vi "RT Main.vi"() -> ()   [LabVIEW 2013]
uses:
  SubVIs/growbed_states.ctl
  SubVIs/fishtank_level_states.ctl
  SubVIs/fishtank_states.ctl
  <vilib>/Platform/TimedLoop/XDataNode/timing_clust.ctl
  <vilib>/Platform/TimedLoop/XDataNode/nitl_modes.ctl
  <vilib>/Platform/TimedLoop/XDataNode/wakeup.ctl
  SubVIs/FGV_enum.ctl
  <vilib>/rvi/interface/common/niFpgaWaitOnOcc.vi
  <vilib>/FPGAPlugInAG/myRIO-1900/niLvFpga_Open_myRIO-1900.vi
  <vilib>/rvi/interface/common/dynamic/niFpgaDynamicAddResources.vi
  <vilib>/Utility/error.llb/Error Cluster From Error Code.vi
  <vilib>/rvi/errors/niLvFpgaAdjustHostInterfaceError.vi
  <vilib>/FPGAPlugInAG/Dynamic/niLvFpga_Run_Dynamic.vi
  <vilib>/FPGAPlugInAG/Dynamic/niLvFpga_Close_Dynamic.vi
  <vilib>/rvi/interface/nirviOpenFPGA/nirviOpenFPGA.xnode
  FPGA Bitfiles/myRIOAquaponics_FPGATarget_Main(FPGA)_Pb0EBwUZ3xI.lvbitx
  <vilib>/rvi/interface/nirviReadWriteControl/nirviReadWriteControl.xnode
  <vilib>/Platform/TimedLoop/XDataNode/XDataNode.xnode
  <vilib>/rvi/interface/nirviMethod/nirviMethod.xnode
  <vilib>/rvi/interface/nirviCloseFPGA/nirviCloseFPGA.xnode
  <vilib>/Platform/TimedLoop/XDataNode/XDNodeRunTimeDep.lvlib
  NiFpgaLv.dll
  <vilib>/rvi/interface/Simulation/niFpgaSimulationCallBeginRW.vi
  <vilib>/rvi/errors/niLvFpgaMergeErrorWithErrorCode.vi
  <vilib>/FPGAPlugInAG/Dynamic/niLvFpga_ConfigureFifo_Dynamic.vi
  <vilib>/FPGAPlugInAG/Dynamic/niLvFpga_StartFifo_Dynamic.vi
  <vilib>/FPGAPlugInAG/Dynamic/niLvFpga_ReadFifo_Dynamic.vi
  <vilib>/FPGAPlugInAG/Dynamic/niLvFpga_StopFifo_Dynamic.vi
panel:
  out "Fishtank States - Temperature":T1=enum."Low Temperature (Heater ON)"
  out "pH Signal":dbl[](graph)=[0.029296875, 0.0244140625, 0.0244140625, 0.0244140625, 0.01953125, 0.029296875, 0.0244140625, 0.0244140625, 0.0244140625, 0.0244140625, 0.029296875, 0.0244140625, 0.0244140625, 0.029296875, 0.0244140625, 0.029296875, 0.0244140625, 0.0244140625, 0.0244140625, 0.029296875, 0.029296875, 0.0244140625, 0.0244140625, 0.0244140625, 0.029296875, 0.0244140625, 0.0244140625, 0.029296875, 0.0244140625, 0.029296875, 0.029296875, 0.0244140625, 0.029296875, 0.029296875, 0.0244140625, 0.0244140625, 0.0244140625, 0.029296875, 0.029296875, 0.0244140625, 0.029296875, 0.0244140625, 0.029296875, 0.0244140625, 0.029296875, 0.029296875, 0.029296875, 0.0244140625, 0.0244140625, 0.0244140625, 0.0341796875, 0.0244140625, 0.029296875, 0.0244140625, 0.0244140625, 0.029296875, 0.029296875, 0.0341796875, 0.0341796875, 0.0390625, 0.0439453125, 0.0390625, 0.0341796875, 0.0439453125, 0.0439453125, 0.0390625, 0.0439453125, 0.0390625, 0.048828125, 0.0439453125, 0.0390625, 0.0390625, 0.0390625, 0.0439453125, 0.0439453125, 0.0341796875, 0.0439453125, 0.048828125, 0.0390625, 0.048828125, 0.0439453125, 0.048828125, 0.0439453125, 0.0390625, 0.0439453125, 0.0439453125, 0.0439453125, 0.0439453125, 0.0390625, 0.0439453125, 0.0439453125, 0.0439453125, 0.0439453125, 0.0439453125, 0.048828125, 0.048828125, 0.0390625, 0.0439453125, 0.0439453125, 0.0439453125, 0.048828125, 0.0439453125, 0.048828125, 0.048828125, 0.0439453125, 0.048828125, 0.048828125, 0.048828125, 0.048828125, 0.0439453125, 0.048828125, 0.048828125, 0.0390625, 0.048828125, 0.048828125, 0.048828125, 0.048828125, 0.0439453125, 0.048828125, 0.048828125, 0.0439453125, 0.0537109375, 0.048828125, 0.0439453125, 0.048828125, 0.048828125, 0.048828125, 0.0537109375, 0.0439453125, 0.0537109375, 0.048828125, 0.0439453125, 0.048828125, 0.048828125, 0.0439453125, 0.048828125, 0.0439453125, 0.048828125, 0.048828125, 0.048828125, 0.0537109375, 0.048828125, 0.0439453125, 0.0537109375, 0.048828125, 0.0439453125, 0.048828125, 0.0537109375, 0.048828125, 0.0537109375, 0.0439453125, 0.0537109375, 0.048828125, 0.0439453125, 0.05859375, 0.048828125, 0.0439453125, 0.048828125, 0.048828125, 0.048828125, 0.048828125, 0.048828125, 0.048828125, 0.048828125, 0.0439453125, 0.048828125, 0.048828125, 0.048828125, 0.0537109375, 0.048828125, 0.048828125, 0.05859375, 0.048828125, 0.0390625, 0.0537109375, 0.048828125, 0.0439453125, 0.048828125, 0.048828125, 0.048828125, 0.0439453125, 0.048828125, 0.048828125, 0.048828125, 0.0439453125, 0.048828125, 0.048828125, 0.048828125, 0.0537109375, 0.048828125, 0.0439453125, 0.048828125, 0.048828125, 0.048828125, 0.0439453125, 0.048828125, 0.048828125, 0.0439453125, 0.048828125, 0.0537109375, 0.048828125, 0.048828125, 0.048828125, 0.048828125, 0.048828125, 0.0439453125, 0.0537109375, 0.048828125, 0.048828125, 0.0439453125, 0.048828125, 0.048828125, 0.048828125, 0.0537109375, 0.048828125, 0.048828125, 0.0439453125, 0.048828125, 0.048828125, 0.048828125, 0.048828125, 0.0537109375, 0.048828125, 0.0439453125, 0.048828125, 0.048828125, 0.048828125, 0.048828125, 0.048828125, 0.0537109375, 0.048828125, 0.048828125, 0.0390625, 0.048828125, 0.048828125, 0.048828125, 0.048828125, 0.048828125, 0.048828125, 0.0439453125, 0.048828125, 0.048828125, 0.048828125, 0.048828125, 0.0439453125, 0.048828125, 0.0537109375, 0.0439453125, 0.0537109375, 0.048828125, 0.048828125, 0.048828125, 0.0439453125, 0.0537109375, 0.0537109375, 0.0439453125, 0.048828125, 0.048828125, 0.048828125, 0.048828125, 0.048828125, 0.0537109375, 0.048828125, 0.0439453125, 0.0439453125, 0.048828125, 0.0537109375, 0.048828125, 0.0439453125, 0.0439453125, 0.048828125, 0.048828125, 0.048828125, 0.048828125, 0.0537109375, 0.048828125, 0.048828125, 0.0439453125, 0.048828125, 0.0537109375, 0.048828125, 0.0439453125, 0.048828125, 0.048828125, 0.048828125, 0.048828125, 0.0439453125, 0.048828125, 0.048828125, 0.0390625, 0.048828125, 0.0439453125, 0.0439453125, 0.048828125, 0.0439453125, 0.048828125, 0.048828125, 0.0439453125, 0.048828125, 0.0439453125, 0.0439453125, 0.048828125, 0.048828125, 0.048828125, 0.0439453125, 0.048828125, 0.048828125, 0.048828125, 0.0537109375, 0.0439453125, 0.048828125, 0.0439453125, 0.048828125, 0.048828125, 0.0439453125, 0.048828125, 0.0439453125, 0.048828125, 0.048828125, 0.0390625, 0.048828125, 0.0439453125, 0.048828125, 0.048828125, 0.0390625, 0.048828125, 0.048828125, 0.0439453125, 0.0439453125, 0.0439453125, 0.048828125, 0.0439453125, 0.0439453125, 0.0439453125, 0.0390625, 0.048828125, 0.0439453125, 0.0439453125, 0.048828125, 0.0390625, 0.048828125, 0.0390625, 0.0439453125, 0.048828125, 0.0390625, 0.048828125, 0.0390625, 0.0390625, 0.0439453125, 0.0439453125, 0.048828125, 0.0390625, 0.0439453125, 0.0439453125, 0.0439453125, 0.0439453125, 0.0439453125, 0.048828125, 0.0390625, 0.0439453125, 0.0439453125, 0.0390625, 0.048828125, 0.0341796875, 0.0390625, 0.0439453125, 0.0439453125, 0.0439453125, 0.0390625, 0.048828125, 0.0439453125, 0.0390625, 0.0439453125, 0.0439453125, 0.0439453125, 0.0341796875, 0.0390625, 0.0439453125, 0.0439453125, 0.0439453125, 0.0390625, 0.048828125, 0.0439453125, 0.0390625, 0.048828125, 0.0390625, 0.0439453125, 0.0390625, 0.0439453125, 0.0439453125, 0.0390625, 0.0390625, 0.0390625, 0.0439453125, 0.0390625, 0.0439453125, 0.0439453125, 0.0439453125, 0.0439453125, 0.0390625, 0.0390625, 0.0439453125, 0.0439453125, 0.0439453125, 0.0390625, 0.0439453125, 0.0439453125, 0.0390625, 0.0439453125, 0.0390625, 0.0390625, 0.0341796875, 0.0439453125, 0.0439453125, 0.0390625, 0.0439453125, 0.0390625, 0.0439453125, 0.0390625, 0.0439453125, 0.0439453125, 0.0341796875, 0.0439453125, 0.0439453125, 0.0390625, 0.0439453125, 0.0390625, 0.0439453125, 0.0439453125, 0.0439453125, 0.0439453125, 0.0390625, 0.0390625, 0.0341796875, 0.0390625, 0.0439453125, 0.0390625, 0.0439453125, 0.0341796875, 0.0439453125, 0.048828125, 0.0390625, 0.0390625, 0.0341796875, 0.0390625, 0.0439453125, 0.0390625, 0.0390625, 0.0390625, 0.0390625, 0.0390625, 0.0439453125, 0.0439453125, 0.0390625, 0.0390625, 0.0390625, 0.0439453125, 0.0390625, 0.0341796875, 0.0439453125, 0.0439453125, 0.0439453125, 0.0390625, 0.0390625, 0.0390625, 0.0439453125, 0.0439453125, 0.0439453125, 0.0390625, 0.0390625, 0.0439453125, 0.0390625, 0.0439453125, 0.0439453125, 0.0439453125, 0.0390625, 0.0439453125, 0.0390625, 0.0390625, 0.0439453125, 0.0439453125, 0.0439453125, 0.0390625, 0.0439453125, 0.048828125, 0.0390625, 0.0390625, 0.0390625, 0.0390625, 0.0439453125, 0.0439453125, 0.0439453125, 0.048828125, 0.0390625, 0.0390625, 0.0390625, 0.0439453125, 0.0439453125, 0.0439453125, 0.0390625, 0.0390625, 0.0439453125, 0.0439453125, 0.0439453125, 0.0439453125, 0.0439453125, 0.0439453125, 0.0390625, 0.0390625, 0.0439453125, 0.0439453125, 0.0439453125, 0.0439453125, 0.0439453125, 0.0439453125, 0.0390625, 0.0390625, 0.0439453125, 0.0439453125, 0.0390625, 0.0439453125, 0.0439453125, 0.0390625, 0.0439453125, 0.0390625, 0.0439453125, 0.0439453125, 0.0390625, 0.0439453125, 0.0439453125, 0.0439453125, 0.0439453125, 0.0390625, 0.0439453125, 0.0439453125, 0.0439453125, 0.0439453125, 0.0439453125, 0.0439453125, 0.0439453125, 0.0390625, 0.0439453125, 0.0439453125, 0.0390625, 0.0439453125, 0.048828125, 0.0390625, 0.0439453125, 0.0439453125, 0.0390625, 0.0439453125, 0.0390625, 0.0439453125, 0.048828125, 0.0390625, 0.0390625, 0.048828125, 0.0390625, 0.0439453125, 0.048828125, 0.0390625, 0.0390625, 0.0390625, 0.0439453125, 0.0439453125, 0.0390625, 0.0390625, 0.0439453125, 0.0390625, 0.0390625, 0.048828125, 0.0439453125, 0.0390625, 0.0439453125, 0.0390625, 0.0390625, 0.0390625, 0.0390625, 0.048828125, 0.0390625, 0.0390625, 0.0439453125, 0.0390625, 0.0390625, 0.0439453125, 0.0390625, 0.048828125, 0.0439453125, 0.0439453125, 0.0390625, 0.0439453125, 0.0390625, 0.0390625, 0.0439453125, 0.0390625, 0.0439453125, 0.0390625, 0.0439453125, 0.0439453125, 0.0341796875, 0.0439453125, 0.0439453125, 0.0439453125, 0.0390625, 0.0439453125, 0.0390625, 0.0439453125, 0.0439453125, 0.0439453125, 0.0390625, 0.0390625, 0.0439453125, 0.0390625, 0.0390625, 0.0439453125, 0.0439453125, 0.0390625, 0.0439453125, 0.0439453125, 0.0439453125, 0.0390625, 0.0390625, 0.0439453125, 0.0390625, 0.0390625, 0.0439453125, 0.0439453125, 0.0439453125, 0.0439453125, 0.0439453125, 0.0439453125, 0.0390625, 0.0390625, 0.0439453125, 0.0439453125, 0.0390625, 0.0439453125, 0.0439453125, 0.0390625, 0.0439453125, 0.048828125, 0.0390625, 0.0439453125, 0.0390625, 0.0439453125, 0.0439453125, 0.0439453125, 0.0439453125, 0.0439453125, 0.0439453125, 0.0439453125, 0.0390625, 0.0439453125, 0.0439453125, 0.0390625, 0.0390625, 0.0439453125, 0.0439453125, 0.0390625, 0.0390625, 0.0390625, 0.0439453125, 0.0439453125, 0.0390625, 0.048828125, 0.0390625, 0.0390625, 0.0390625, 0.0439453125, 0.0439453125, 0.0439453125, 0.0439453125, 0.048828125, 0.0439453125, 0.0439453125, 0.0390625, 0.0390625, 0.0439453125, 0.0439453125, 0.0390625, 0.0439453125, 0.0390625, 0.0439453125, 0.0439453125, 0.0390625, 0.0439453125, 0.0439453125, 0.0390625, 0.0390625, 0.0439453125, 0.0439453125, 0.0390625, 0.0390625, 0.0390625, 0.0439453125, 0.0390625, 0.0390625, 0.0439453125, 0.0390625, 0.0390625, 0.0439453125, 0.0390625, 0.0390625, 0.048828125, 0.0439453125, 0.0439453125, 0.0390625, 0.0390625, 0.048828125, 0.0390625, 0.0390625, 0.0390625, 0.0439453125, 0.0439453125, 0.0439453125, 0.0341796875, 0.0390625, 0.0439453125, 0.0439453125, 0.0439453125, 0.0390625, 0.0390625, 0.0439453125, 0.0390625, 0.0439453125, 0.0390625, 0.0390625, 0.0390625, 0.0439453125, 0.0390625, 0.0439453125, 0.0390625, 0.0390625, 0.0439453125, 0.0439453125, 0.0390625, 0.0439453125, 0.0390625, 0.0390625, 0.0390625, 0.0390625, 0.0390625, 0.0439453125, 0.0390625, 0.0439453125, 0.0341796875, 0.0390625, 0.0439453125, 0.0390625, 0.0390625, 0.0390625, 0.0390625, 0.0390625, 0.0439453125, 0.0390625, 0.0439453125, 0.0390625, 0.0390625, 0.0439453125, 0.0390625, 0.0390625, 0.0390625, 0.0390625, 0.0390625, 0.0390625, 0.0390625, 0.0439453125, 0.0439453125, 0.0390625, 0.0439453125, 0.0390625, 0.0390625, 0.0390625, 0.0341796875, 0.0390625, 0.0439453125, 0.0390625, 0.0439453125, 0.0390625, 0.0439453125, 0.0439453125, 0.0390625, 0.0341796875, 0.0439453125, 0.0341796875, 0.0390625, 0.0439453125, 0.0439453125, 0.0390625, 0.0439453125, 0.0390625, 0.0390625, 0.0390625, 0.0390625, 0.0390625, 0.0390625, 0.0390625, 0.0390625, 0.0390625, 0.0439453125, 0.0390625, 0.0390625, 0.0439453125, 0.0390625, 0.0390625, 0.0390625, 0.0390625, 0.0341796875, 0.0390625, 0.0390625, 0.0390625, 0.0439453125, 0.0390625, 0.0390625, 0.0439453125, 0.0390625, 0.0390625, 0.0390625, 0.0390625, 0.0390625, 0.0341796875, 0.0341796875, 0.0390625, 0.0390625, 0.0390625, 0.0390625, 0.0341796875, 0.0390625, 0.0439453125, 0.0341796875, 0.0390625, 0.0390625, 0.0390625, 0.0390625, 0.0390625, 0.0390625, 0.0390625, 0.0341796875, 0.0390625, 0.0439453125, 0.0439453125, 0.0390625, 0.0390625, 0.0341796875, 0.0390625, 0.0390625, 0.0390625, 0.0390625, 0.0341796875, 0.0341796875, 0.0439453125, 0.0390625, 0.0390625, 0.0341796875, 0.0341796875, 0.0439453125, 0.0341796875, 0.0390625, 0.0390625, 0.0390625, 0.0390625, 0.0341796875, 0.0390625, 0.0439453125, 0.0390625, 0.0390625, 0.0390625, 0.0341796875, 0.0390625, 0.0390625, 0.0390625, 0.0341796875, 0.0390625, 0.0390625, 0.0390625, 0.0439453125, 0.0341796875, 0.0390625, 0.0341796875, 0.0341796875, 0.0390625, 0.029296875, 0.0244140625, 0.0244140625, 0.0244140625, 0.01953125, 0.029296875, 0.01953125, 0.01953125, 0.0244140625, 0.01953125, 0.029296875, 0.0146484375, 0.01953125, 0.029296875, 0.01953125, 0.0244140625, 0.01953125, 0.01953125, 0.0244140625, 0.01953125, 0.01953125, 0.0244140625, 0.01953125, 0.0244140625, 0.01953125, 0.0146484375, 0.0244140625, 0.01953125, 0.01953125, 0.01953125, 0.0146484375, 0.01953125, 0.0146484375, 0.01953125, 0.01953125, 0.01953125, 0.0244140625, 0.0146484375, 0.0146484375, 0.01953125, 0.0146484375, 0.01953125, 0.01953125, 0.0146484375, 0.01953125, 0.0146484375, 0.01953125, 0.0146484375, 0.0146484375, 0.0244140625, 0.0146484375, 0.009765625, 0.01953125, 0.0146484375, 0.01953125, 0.0146484375, 0.0146484375, 0.0244140625, 0.009765625, 0.009765625, 0.01953125, 0.0146484375, 0.0146484375, 0.0146484375, 0.0146484375, 0.01953125, 0.0146484375, 0.009765625, 0.01953125, 0.009765625, 0.009765625, 0.01953125, 0.009765625, 0.01953125, 0.01953125, 0.0146484375, 0.01953125, 0.009765625, 0.0146484375, 0.01953125, 0.009765625, 0.0146484375, 0.0146484375, 0.009765625, 0.01953125, 0.009765625, 0.009765625, 0.0146484375, 0.009765625, 0.0146484375, 0.01953125, 0.009765625, 0.0146484375, 0.0146484375, 0.009765625, 0.0146484375, 0.0146484375, 0.0146484375, 0.0146484375, 0.009765625, 0.009765625, 0.01953125, 0.009765625, 0.0146484375, 0.0146484375, 0.009765625, 0.0146484375, 0.0146484375, 0.0146484375, 0.01953125, 0.009765625, 0.0146484375, 0.0146484375, 0.009765625, 0.009765625, 0.01953125, 0.009765625, 0.009765625, 0.0146484375, 0.009765625, 0.0146484375, 0.01953125, 0.009765625, 0.0146484375, 0.0146484375, 0.0146484375, 0.01953125, 0.0146484375, 0.0146484375, 0.01953125, 0.0048828125, 0.0146484375, 0.01953125, 0.009765625, 0.009765625, 0.01953125, 0.009765625, 0.0146484375, 0.0146484375, 0.009765625, 0.0146484375, 0.0146484375, 0.009765625, 0.01953125, 0.009765625, 0.0146484375, 0.0146484375, 0.009765625, 0.0146484375, 0.01953125, 0.009765625, 0.0146484375, 0.0146484375, 0.009765625, 0.01953125, 0.0146484375, 0.0146484375, 0.01953125, 0.009765625, 0.009765625, 0.01953125, 0.009765625, 0.0146484375, 0.01953125, 0.009765625, 0.0146484375, 0.0146484375, 0.0146484375, 0.01953125, 0.0048828125, 0.009765625, 0.01953125, 0.009765625, 0.01953125, 0.0146484375, 0.0146484375, 0.01953125, 0.0048828125, 0.009765625, 0.0146484375, 0.009765625, 0.0146484375, 0.0146484375, 0.009765625, 0.0146484375, 0.0146484375, 0.0146484375, 0.01953125, 0.0146484375, 0.009765625, 0.01953125, 0.009765625, 0.0146484375, 0.0244140625, 0.0146484375, 0.0146484375, 0.0146484375, 0.0048828125, 0.01953125, 0.0146484375, 0.009765625, 0.009765625, 0.009765625, 0.0146484375, 0.009765625, 0.009765625, 0.0146484375, 0.0146484375, 0.0146484375, 0.009765625, 0.0146484375, 0.0146484375, 0.0146484375, 0.0146484375, 0.0146484375, 0.01953125, 0.01953125, 0.009765625, 0.0146484375, 0.01953125, 0.0146484375, 0.0146484375, 0.0146484375, 0.0146484375, 0.0146484375, 0.009765625, 0.01953125, 0.0146484375, 0.0146484375, 0.01953125, 0.009765625, 0.009765625, 0.0146484375, 0.009765625, 0.0146484375, 0.009765625, 0.009765625, 0.01953125, 0.009765625, 0.0146484375, 0.0146484375, 0.0146484375, 0.01953125, 0.0146484375, 0.01953125, 0.0244140625, 0.0244140625, 0.01953125, 0.01953125, 0.01953125, 0.01953125, 0.0244140625, 0.0244140625, 0.01953125, 0.01953125, 0.0244140625, 0.0244140625, 0.0244140625, 0.01953125, 0.01953125, 0.0244140625, 0.0244140625, 0.0244140625, 0.0146484375, 0.01953125, 0.0244140625, 0.01953125, 0.0244140625, 0.0146484375, 0.01953125, 0.0244140625, 0.0244140625, 0.0244140625, 0.01953125, 0.01953125, 0.01953125, 0.0244140625, 0.029296875, 0.01953125, 0.0244140625, 0.01953125, 0.0244140625, 0.029296875, 0.01953125, 0.0244140625, 0.01953125, 0.0244140625, 0.029296875, 0.01953125, 0.0244140625, 0.0244140625, 0.01953125, 0.01953125, 0.01953125, 0.0244140625, 0.0244140625, 0.01953125, 0.0244140625, 0.0244140625, 0.0244140625, 0.0146484375, 0.01953125, 0.0244140625, 0.0244140625, 0.0244140625, 0.01953125, 0.01953125, 0.0244140625, 0.01953125, 0.0244140625, 0.01953125, 0.0244140625, 0.0244140625, 0.01953125, 0.0244140625, 0.01953125, 0.01953125, 0.0146484375, 0.01953125, 0.0244140625, 0.0244140625, 0.0244140625, 0.01953125, 0.0244140625, 0.01953125, 0.0244140625, 0.0244140625, 0.01953125, 0.0244140625, 0.01953125, 0.01953125, 0.0244140625, 0.0244140625, 0.0244140625, 0.0244140625, 0.0244140625, 0.0244140625, 0.01953125, 0.0244140625, 0.01953125, 0.0244140625, 0.01953125, 0.01953125, 0.01953125, 0.0244140625, 0.029296875, 0.01953125, 0.0244140625, 0.01953125, 0.01953125, 0.0244140625, 0.0244140625, 0.0244140625, 0.0146484375, 0.01953125, 0.01953125, 0.029296875, 0.0244140625, 0.01953125, 0.0244140625, 0.0244140625, 0.0244140625, 0.0244140625, 0.01953125, 0.029296875, 0.01953125, 0.01953125, 0.0244140625, 0.0244140625, 0.0244140625, 0.01953125, 0.0146484375, 0.01953125, 0.0244140625, 0.029296875, 0.0146484375, 0.0244140625, 0.0244140625, 0.0244140625, 0.0244140625, 0.01953125, 0.029296875, 0.01953125, 0.01953125, 0.029296875, 0.01953125, 0.029296875, 0.01953125, 0.01953125, 0.0244140625, 0.01953125, 0.0244140625, 0.01953125, 0.01953125, 0.0244140625, 0.0244140625, 0.01953125, 0.01953125, 0.0244140625, 0.01953125, 0.0244140625, 0.0244140625, 0.01953125, 0.01953125, 0.0244140625, 0.0244140625, 0.0244140625, 0.01953125, 0.01953125, 0.0244140625, 0.0244140625, 0.0244140625, 0.0244140625, 0.01953125, 0.01953125, 0.0244140625, 0.0244140625, 0.0244140625, 0.01953125, 0.01953125, 0.0244140625, 0.0244140625, 0.0244140625, 0.0244140625, 0.01953125, 0.01953125, 0.01953125, 0.01953125, 0.029296875, 0.0244140625, 0.01953125, 0.0244140625, 0.01953125, 0.0244140625, 0.01953125, 0.0146484375, 0.01953125, 0.0244140625, 0.0244140625, 0.0244140625, 0.0244140625, 0.0244140625, 0.01953125, 0.0244140625, 0.01953125, 0.01953125, 0.0244140625, 0.01953125, 0.0244140625, 0.01953125, 0.0244140625, 0.0244140625, 0.01953125, 0.0244140625, 0.01953125, 0.01953125, 0.0244140625, 0.0146484375, 0.01953125, 0.0244140625, 0.0244140625, 0.01953125, 0.0244140625, 0.0244140625, 0.0244140625, 0.01953125, 0.0146484375, 0.0244140625, 0.0244140625, 0.01953125, 0.01953125, 0.01953125, 0.01953125, 0.0244140625, 0.0244140625, 0.0244140625, 0.0244140625, 0.01953125, 0.01953125, 0.01953125, 0.0244140625, 0.0244140625, 0.01953125, 0.0244140625, 0.0244140625, 0.0146484375, 0.0244140625, 0.01953125, 0.01953125, 0.01953125, 0.0146484375, 0.0244140625, 0.0244140625, 0.01953125, 0.0244140625, 0.0244140625, 0.0244140625, 0.0146484375, 0.0244140625, 0.01953125, 0.0244140625, 0.01953125, 0.0244140625, 0.0244140625, 0.0146484375, 0.01953125, 0.0244140625, 0.0244140625, 0.01953125, 0.01953125, 0.0244140625, 0.01953125, 0.0244140625, 0.0244140625, 0.0244140625, 0.01953125, 0.01953125, 0.01953125, 0.0244140625, 0.01953125, 0.0244140625, 0.01953125, 0.01953125, 0.0244140625, 0.0244140625, 0.01953125, 0.01953125, 0.0244140625, 0.0244140625, 0.0146484375, 0.0244140625, 0.01953125, 0.01953125, 0.0146484375, 0.0244140625, 0.0244140625, 0.01953125, 0.01953125, 0.01953125, 0.0244140625, 0.0244140625, 0.0244140625, 0.01953125, 0.0244140625, 0.0244140625, 0.0244140625, 0.01953125, 0.029296875, 0.01953125, 0.01953125, 0.0244140625, 0.01953125, 0.01953125, 0.01953125, 0.01953125, 0.0244140625, 0.01953125, 0.01953125, 0.0244140625, 0.01953125, 0.0244140625, 0.0244140625, 0.01953125, 0.01953125, 0.01953125, 0.01953125, 0.0244140625, 0.0244140625, 0.01953125, 0.01953125, 0.0244140625, 0.01953125, 0.029296875, 0.01953125, 0.01953125, 0.029296875, 0.01953125, 0.01953125, 0.01953125, 0.0244140625, 0.0244140625, 0.01953125, 0.01953125, 0.0244140625, 0.01953125, 0.01953125, 0.0244140625, 0.01953125, 0.01953125, 0.01953125, 0.01953125, 0.0244140625, 0.01953125, 0.01953125, 0.0244140625, 0.0244140625, 0.0146484375, 0.01953125, 0.01953125, 0.0244140625, 0.01953125, 0.01953125, 0.0244140625, 0.0244140625, 0.0146484375, 0.01953125, 0.01953125, 0.0244140625, 0.01953125, 0.0244140625, 0.0244140625, 0.0244140625, 0.01953125, 0.01953125, 0.0244140625, 0.0244140625, 0.01953125, 0.0244140625, 0.0244140625, 0.0244140625, 0.0146484375, 0.01953125, 0.0244140625, 0.01953125, 0.01953125, 0.0244140625, 0.0244140625, 0.0244140625, 0.01953125, 0.01953125, 0.0244140625, 0.0244140625, 0.01953125, 0.0244140625, 0.0244140625, 0.01953125, 0.0244140625, 0.01953125, 0.01953125, 0.0244140625, 0.01953125, 0.01953125, 0.01953125, 0.01953125, 0.0244140625, 0.01953125, 0.01953125, 0.0244140625, 0.01953125, 0.0244140625, 0.0244140625, 0.01953125, 0.029296875, 0.0244140625, 0.0244140625, 0.01953125, 0.01953125, 0.0244140625, 0.0244140625, 0.01953125, 0.01953125, 0.0244140625, 0.0244140625, 0.01953125, 0.01953125, 0.01953125, 0.0244140625, 0.01953125, 0.01953125, 0.0244140625, 0.01953125, 0.0244140625, 0.0244140625, 0.01953125, 0.0244140625, 0.01953125, 0.01953125, 0.0244140625, 0.0244140625, 0.01953125, 0.0244140625, 0.01953125, 0.0244140625, 0.0244140625, 0.0244140625, 0.01953125, 0.01953125, 0.01953125, 0.0244140625, 0.0244140625, 0.01953125, 0.0244140625, 0.0244140625, 0.01953125, 0.0244140625, 0.0146484375, 0.0244140625, 0.0244140625, 0.01953125, 0.01953125, 0.0244140625, 0.0244140625, 0.0244140625, 0.01953125, 0.01953125, 0.01953125, 0.0244140625, 0.01953125, 0.0244140625, 0.01953125, 0.01953125, 0.01953125, 0.0244140625, 0.0244140625, 0.01953125, 0.0146484375, 0.0244140625, 0.029296875, 0.01953125, 0.0244140625, 0.0244140625, 0.0244140625, 0.0244140625, 0.01953125, 0.0244140625, 0.01953125, 0.01953125, 0.01953125, 0.0244140625, 0.0244140625, 0.0244140625, 0.01953125, 0.01953125, 0.0244140625, 0.029296875, 0.0244140625, 0.0244140625, 0.0244140625, 0.0244140625, 0.01953125, 0.0244140625, 0.029296875, 0.0244140625, 0.01953125, 0.01953125, 0.01953125, 0.029296875, 0.0244140625, 0.0244140625, 0.0244140625, 0.0244140625, 0.01953125, 0.029296875, 0.029296875, 0.01953125, 0.0244140625, 0.01953125, 0.0244140625, 0.0244140625, 0.01953125, 0.0244140625, 0.029296875, 0.01953125, 0.0244140625, 0.0244140625, 0.029296875, 0.0244140625, 0.0244140625, 0.01953125, 0.0244140625, 0.0244140625, 0.0244140625, 0.0244140625, 0.0244140625, 0.01953125, 0.0244140625, 0.0244140625, 0.029296875, 0.0244140625, 0.01953125, 0.01953125, 0.01953125, 0.0244140625, 0.029296875, 0.0244140625, 0.0244140625, 0.0244140625, 0.0244140625, 0.0244140625, 0.029296875, 0.0244140625, 0.029296875, 0.01953125, 0.0244140625, 0.0244140625, 0.0244140625, 0.01953125, 0.0244140625, 0.0244140625, 0.029296875, 0.0244140625, 0.0244140625, 0.0244140625, 0.0244140625, 0.0244140625, 0.029296875, 0.01953125, 0.0244140625, 0.029296875, 0.029296875, 0.0244140625, 0.029296875, 0.01953125, 0.0244140625, 0.029296875, 0.029296875, 0.0244140625, 0.01953125, 0.0244140625, 0.0341796875, 0.029296875, 0.0244140625, 0.01953125, 0.0244140625, 0.029296875, 0.029296875, 0.0244140625, 0.0244140625, 0.0244140625, 0.0244140625, 0.029296875, 0.0244140625, 0.0244140625, 0.0244140625, 0.029296875, 0.029296875, 0.0244140625, 0.01953125, 0.029296875, 0.0244140625, 0.0244140625, 0.0244140625, 0.029296875, 0.0390625, 0.0390625, 0.0390625, 0.0390625, 0.0390625, 0.0390625, 0.0390625, 0.0439453125, 0.0390625, 0.048828125, 0.0390625, 0.0390625, 0.0439453125, 0.0341796875, 0.0439453125, 0.0439453125, 0.0341796875, 0.0439453125, 0.0439453125, 0.0439453125, 0.0439453125, 0.0439453125, 0.0439453125, 0.0439453125, 0.0439453125, 0.0390625, 0.0439453125, 0.0439453125, 0.0439453125, 0.0390625, 0.0439453125, 0.048828125, 0.0439453125, 0.0439453125, 0.048828125, 0.048828125, 0.048828125, 0.0439453125, 0.0439453125, 0.048828125, 0.048828125, 0.0439453125, 0.048828125, 0.048828125, 0.048828125, 0.0439453125, 0.0439453125, 0.0439453125, 0.048828125, 0.0439453125, 0.0439453125, 0.048828125, 0.0439453125, 0.0439453125, 0.048828125, 0.048828125, 0.048828125, 0.0439453125, 0.0439453125, 0.0537109375, 0.048828125, 0.0439453125, 0.048828125, 0.048828125, 0.048828125, 0.048828125, 0.048828125, 0.0537109375, 0.048828125, 0.0390625, 0.048828125, 0.048828125, 0.048828125, 0.0537109375, 0.048828125, 0.048828125, 0.048828125, 0.048828125, 0.0537109375, 0.0537109375, 0.0439453125, 0.048828125, 0.048828125, 0.048828125, 0.048828125, 0.0439453125, 0.0537109375, 0.048828125, 0.0439453125, 0.0537109375, 0.0537109375, 0.0439453125, 0.0537109375, 0.0439453125, 0.048828125, 0.048828125, 0.048828125, 0.048828125, 0.048828125, 0.048828125, 0.048828125, 0.0537109375, 0.048828125, 0.05859375, 0.048828125, 0.0439453125, 0.048828125, 0.048828125, 0.048828125, 0.048828125, 0.048828125, 0.048828125, 0.048828125, 0.0439453125, 0.0537109375, 0.0537109375, 0.048828125, 0.0537109375, 0.048828125, 0.048828125, 0.0537109375, 0.0537109375, 0.0439453125, 0.0537109375, 0.048828125, 0.0439453125, 0.048828125, 0.048828125, 0.048828125, 0.0439453125, 0.048828125, 0.048828125, 0.048828125, 0.048828125, 0.0537109375, 0.0439453125, 0.048828125, 0.0537109375, 0.0537109375, 0.0439453125, 0.0439453125, 0.048828125, 0.048828125, 0.048828125, 0.048828125, 0.048828125, 0.048828125, 0.048828125, 0.0537109375, 0.048828125, 0.048828125, 0.0537109375, 0.0439453125, 0.048828125, 0.048828125, 0.048828125, 0.048828125, 0.048828125, 0.048828125, 0.0537109375, 0.048828125, 0.0439453125, 0.048828125, 0.048828125, 0.048828125, 0.0439453125, 0.0439453125, 0.048828125, 0.048828125, 0.048828125, 0.0537109375, 0.048828125, 0.0439453125, 0.048828125, 0.048828125, 0.0439453125, 0.0439453125, 0.0439453125, 0.05859375, 0.0439453125, 0.0439453125, 0.048828125, 0.048828125, 0.048828125, 0.0537109375, 0.048828125, 0.05859375, 0.0537109375, 0.0439453125, 0.048828125, 0.048828125, 0.048828125, 0.0537109375, 0.048828125, 0.0537109375, 0.0537109375, 0.0439453125, 0.048828125, 0.0537109375, 0.0439453125, 0.048828125, 0.048828125, 0.048828125, 0.048828125, 0.0439453125, 0.048828125, 0.048828125, 0.048828125, 0.048828125, 0.0439453125, 0.048828125, 0.048828125, 0.048828125, 0.0537109375, 0.048828125, 0.0537109375, 0.048828125, 0.048828125, 0.048828125, 0.0439453125, 0.0537109375, 0.048828125, 0.0439453125, 0.048828125, 0.048828125, 0.0537109375, 0.048828125, 0.0439453125, 0.048828125, 0.048828125, 0.048828125, 0.048828125, 0.0439453125, 0.048828125, 0.0439453125, 0.0390625, 0.0439453125, 0.0439453125, 0.048828125, 0.048828125, 0.0439453125, 0.0439453125, 0.0439453125, 0.0439453125, 0.048828125, 0.048828125, 0.0439453125, 0.048828125, 0.048828125, 0.048828125, 0.0439453125, 0.0390625, 0.048828125, 0.0439453125, 0.048828125, 0.0390625, 0.0439453125, 0.048828125, 0.0439453125, 0.048828125, 0.0390625, 0.0439453125, 0.048828125, 0.0439453125, 0.048828125, 0.0390625, 0.0439453125, 0.048828125, 0.0439453125, 0.048828125, 0.0390625, 0.0439453125, 0.0439453125, 0.0439453125, 0.048828125, 0.0439453125]
  out "PH measurement 2":dbl=5.786605646573286
  out "Boolean":bool
  out "Drain - Elapsed Time":dbl=1.1000000000011001e-05
  out "Fish Tank State - Water Level":T2
  out "Pump OFF:\nElapsed Time (s)":dbl
  in  "System Parameters":enum32{"Grow bed", "Fish tank"}(tab)=enum."Fish tank"
  in  "Growbed Flood Level (in) - Fl":dbl=7.4 step=0.05 format="%_4g"
  in  "Flood Level Time (s) - Ft":dbl=10.0 step=0.05 format="%_2g"
  in  "Pump OFF Time (s) - Pt":dbl=15.0 step=0.05 format="%_2g"
  in  "Fish tank Temperature\nThreshold (F) - T1":dbl=88.0 step=0.05 format="%_4g"
  in  "Fish tank minimum\nWater Level (in) - Ml":dbl=2.0 step=0.05 format="%_3g"
  out "Fishtank Distance to H20":dbl=6.015930269449104 format="%0.9f"
  out "Low Water: Elapsed Time (s)":dbl
  out "Growbed State":T3=enum."FLOOD (Pump ON)"
  out "Flood Level: \nElapsed Time (s)":dbl
  out "Growbed Distance to H20":dbl=12.494624405778909 format="%0.9f"
  out "Fishtank: Low Water":bool
  out "Heater On/Off":bool=TRUE
  out "Pump On/Off":bool=TRUE
  out "Fishtank pH Meter - PH1":dbl(knob)=5.786605646573286 scale=1.0..10.0
  out "Growbed Water Level (in) - UTR1":dbl(slide)=4.505375594221091 scale=0.0..10.0
  out "Flowmeter Freq. (Hz)":dbl=25.127501128643594
  out "Flow Rate (L/min)":dbl(knob)=4.56863656884429 caption="Flow Rate (L/min) -\n FLW1" scale=0.0..10.0 scale format="%#_4p"
  out "Fish Tank \nWaterTemperature (F) - TMP1":dbl(slide)=86.7874984741211 scale=-5.0..105.0
  out "Fish Tank\nWater Level (in) -UTR2":dbl(slide)=8.684069730550895 scale=0.0..12.0
  out "Temperature (Graph)":sgl(graph)=30.4375
  in  "Stop Button":bool
  # "myRIO Aquaponics"
  # "Debug Area:"
  # "Overview: Aquaponics Test Panel\nRequirements: LabVIEW FPGA Module.\nInstructions:\n1. Check the myRIO target IP Address in the project and make sure the target IP Address is correct. \n2. Run the VI."
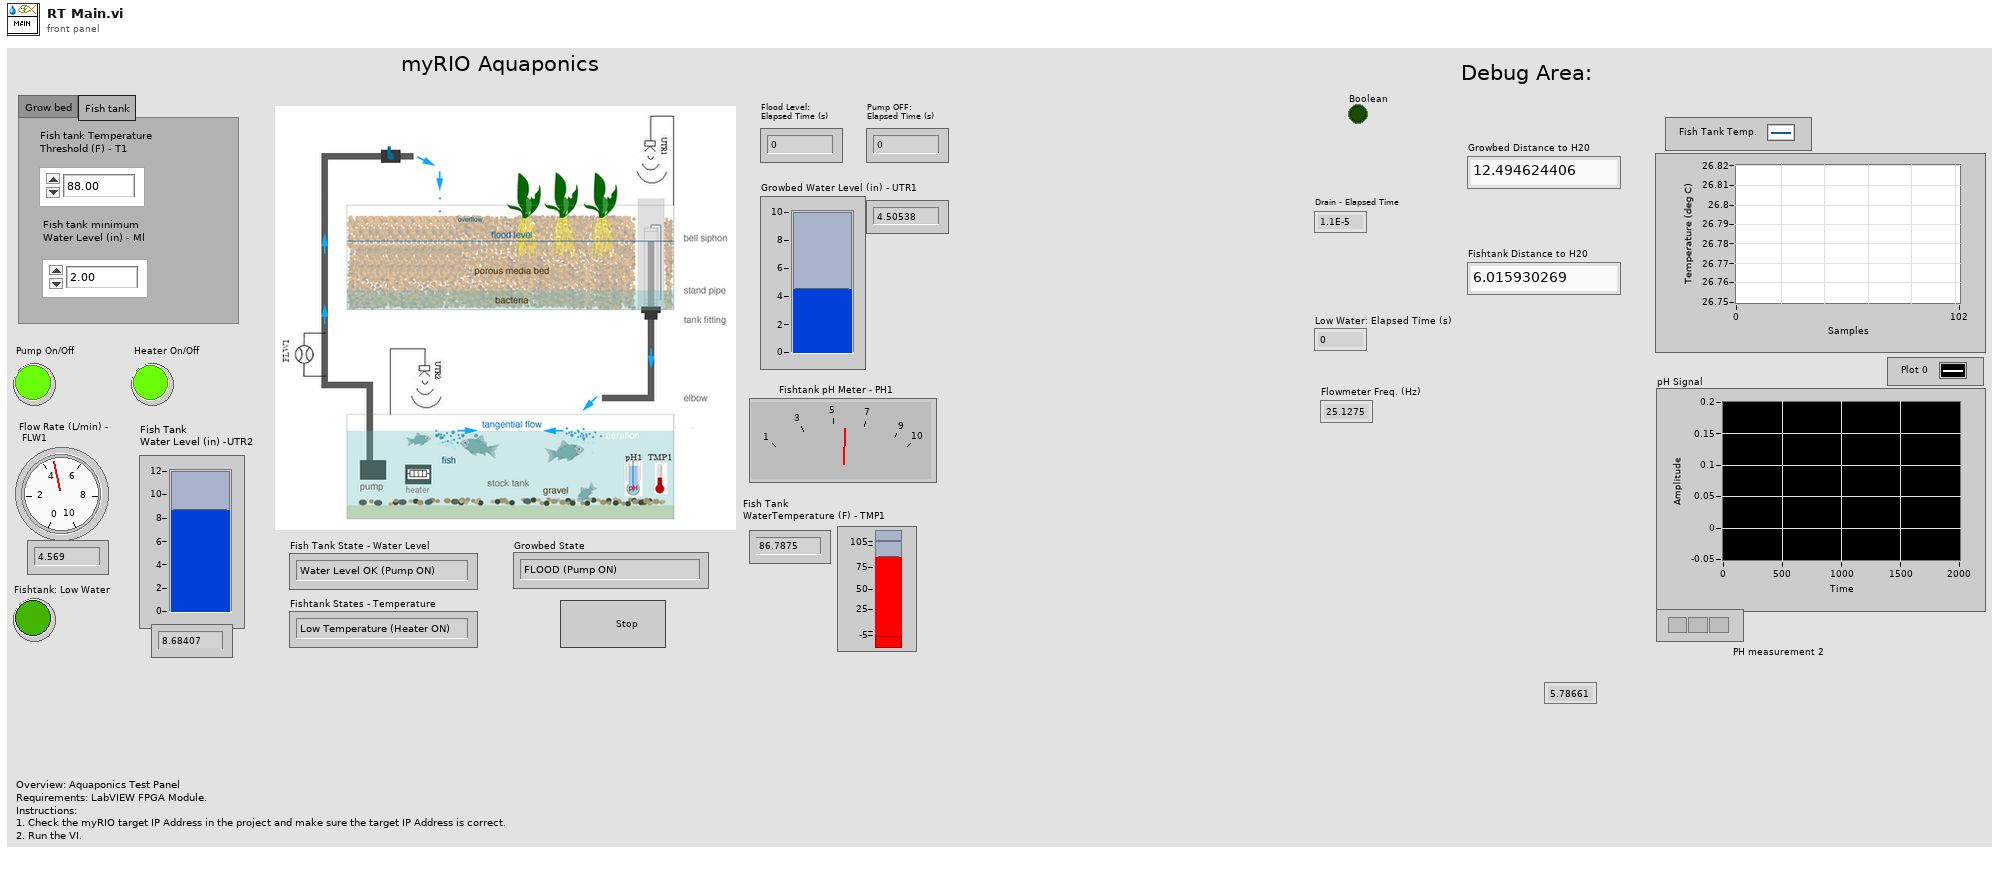
[diagram p1: front panel]
types:
  T1 = typedef "fishtank_states.ctl" = enum16{"Temperature OK (Heater OFF)", "Low Temperature (Heater ON)"}
  T2 = typedef "fishtank_level_states.ctl" = enum16{"Water Level OK (Pump ON)", "Low Water (Pump OFF)"}
  T3 = typedef "growbed_states.ctl" = enum16{"DRAIN (Pump ON)", "FLOOD (Pump ON)", "POST-FLOOD (Pump OFF)", "Low Water - Idle (Pump OFF)", "POST-DRAIN (Pump OFF)"}
  T4 = typedef "XDNodeRunTimeDep.lvlib/timing_clust.ctl" = cluster{"Expected End [f-1]":u64, "Actual End [f-1]":u64, "Finished Late? [f-1]":bool, "Expected End [i-1]":u64, "Actual End [i-1]":u64, "Finished Late? [i-1]":bool, "Expected Start [i]":u64, "Actual Start [i]":u64, "Expected Start [f]":u64, "Actual Start [f]":u64, "Source Name":string, "Structure Name":string, "Period":i64, "Deadline":i64, "Offset":i64, "Start":i64, "Priority":i32, "Timeout":i32, "Mode":T5, "Wakeup Reason":T6, "Error":errorcluster, "Source Type":string, "Secondary Source Type":string, "Global End Time":u64, "Global Start Time":u64, "Frame Duration":u64, "Iteration Duration":u64, "Assigned CPU":i32, "I/O Scan Engine Mode":u32}
  T5 = typedef "XDNodeRunTimeDep.lvlib/nitl_modes.ctl" = enum32{"No Change", "Process missed periods, maintain original phase", "Discard missed periods, maintain original phase", "Process missed periods, ignore original phase", "Discard missed periods, ignore original phase"}
  T6 = typedef "XDNodeRunTimeDep.lvlib/wakeup.ctl" = enum32{"Normal", "Aborted", "Asynchronous wakeup", "Timing source error", "Timed loop error", "Timeout"}
  T7 = typedef "FGV_enum.ctl" = enum16{"Get", "Set"}
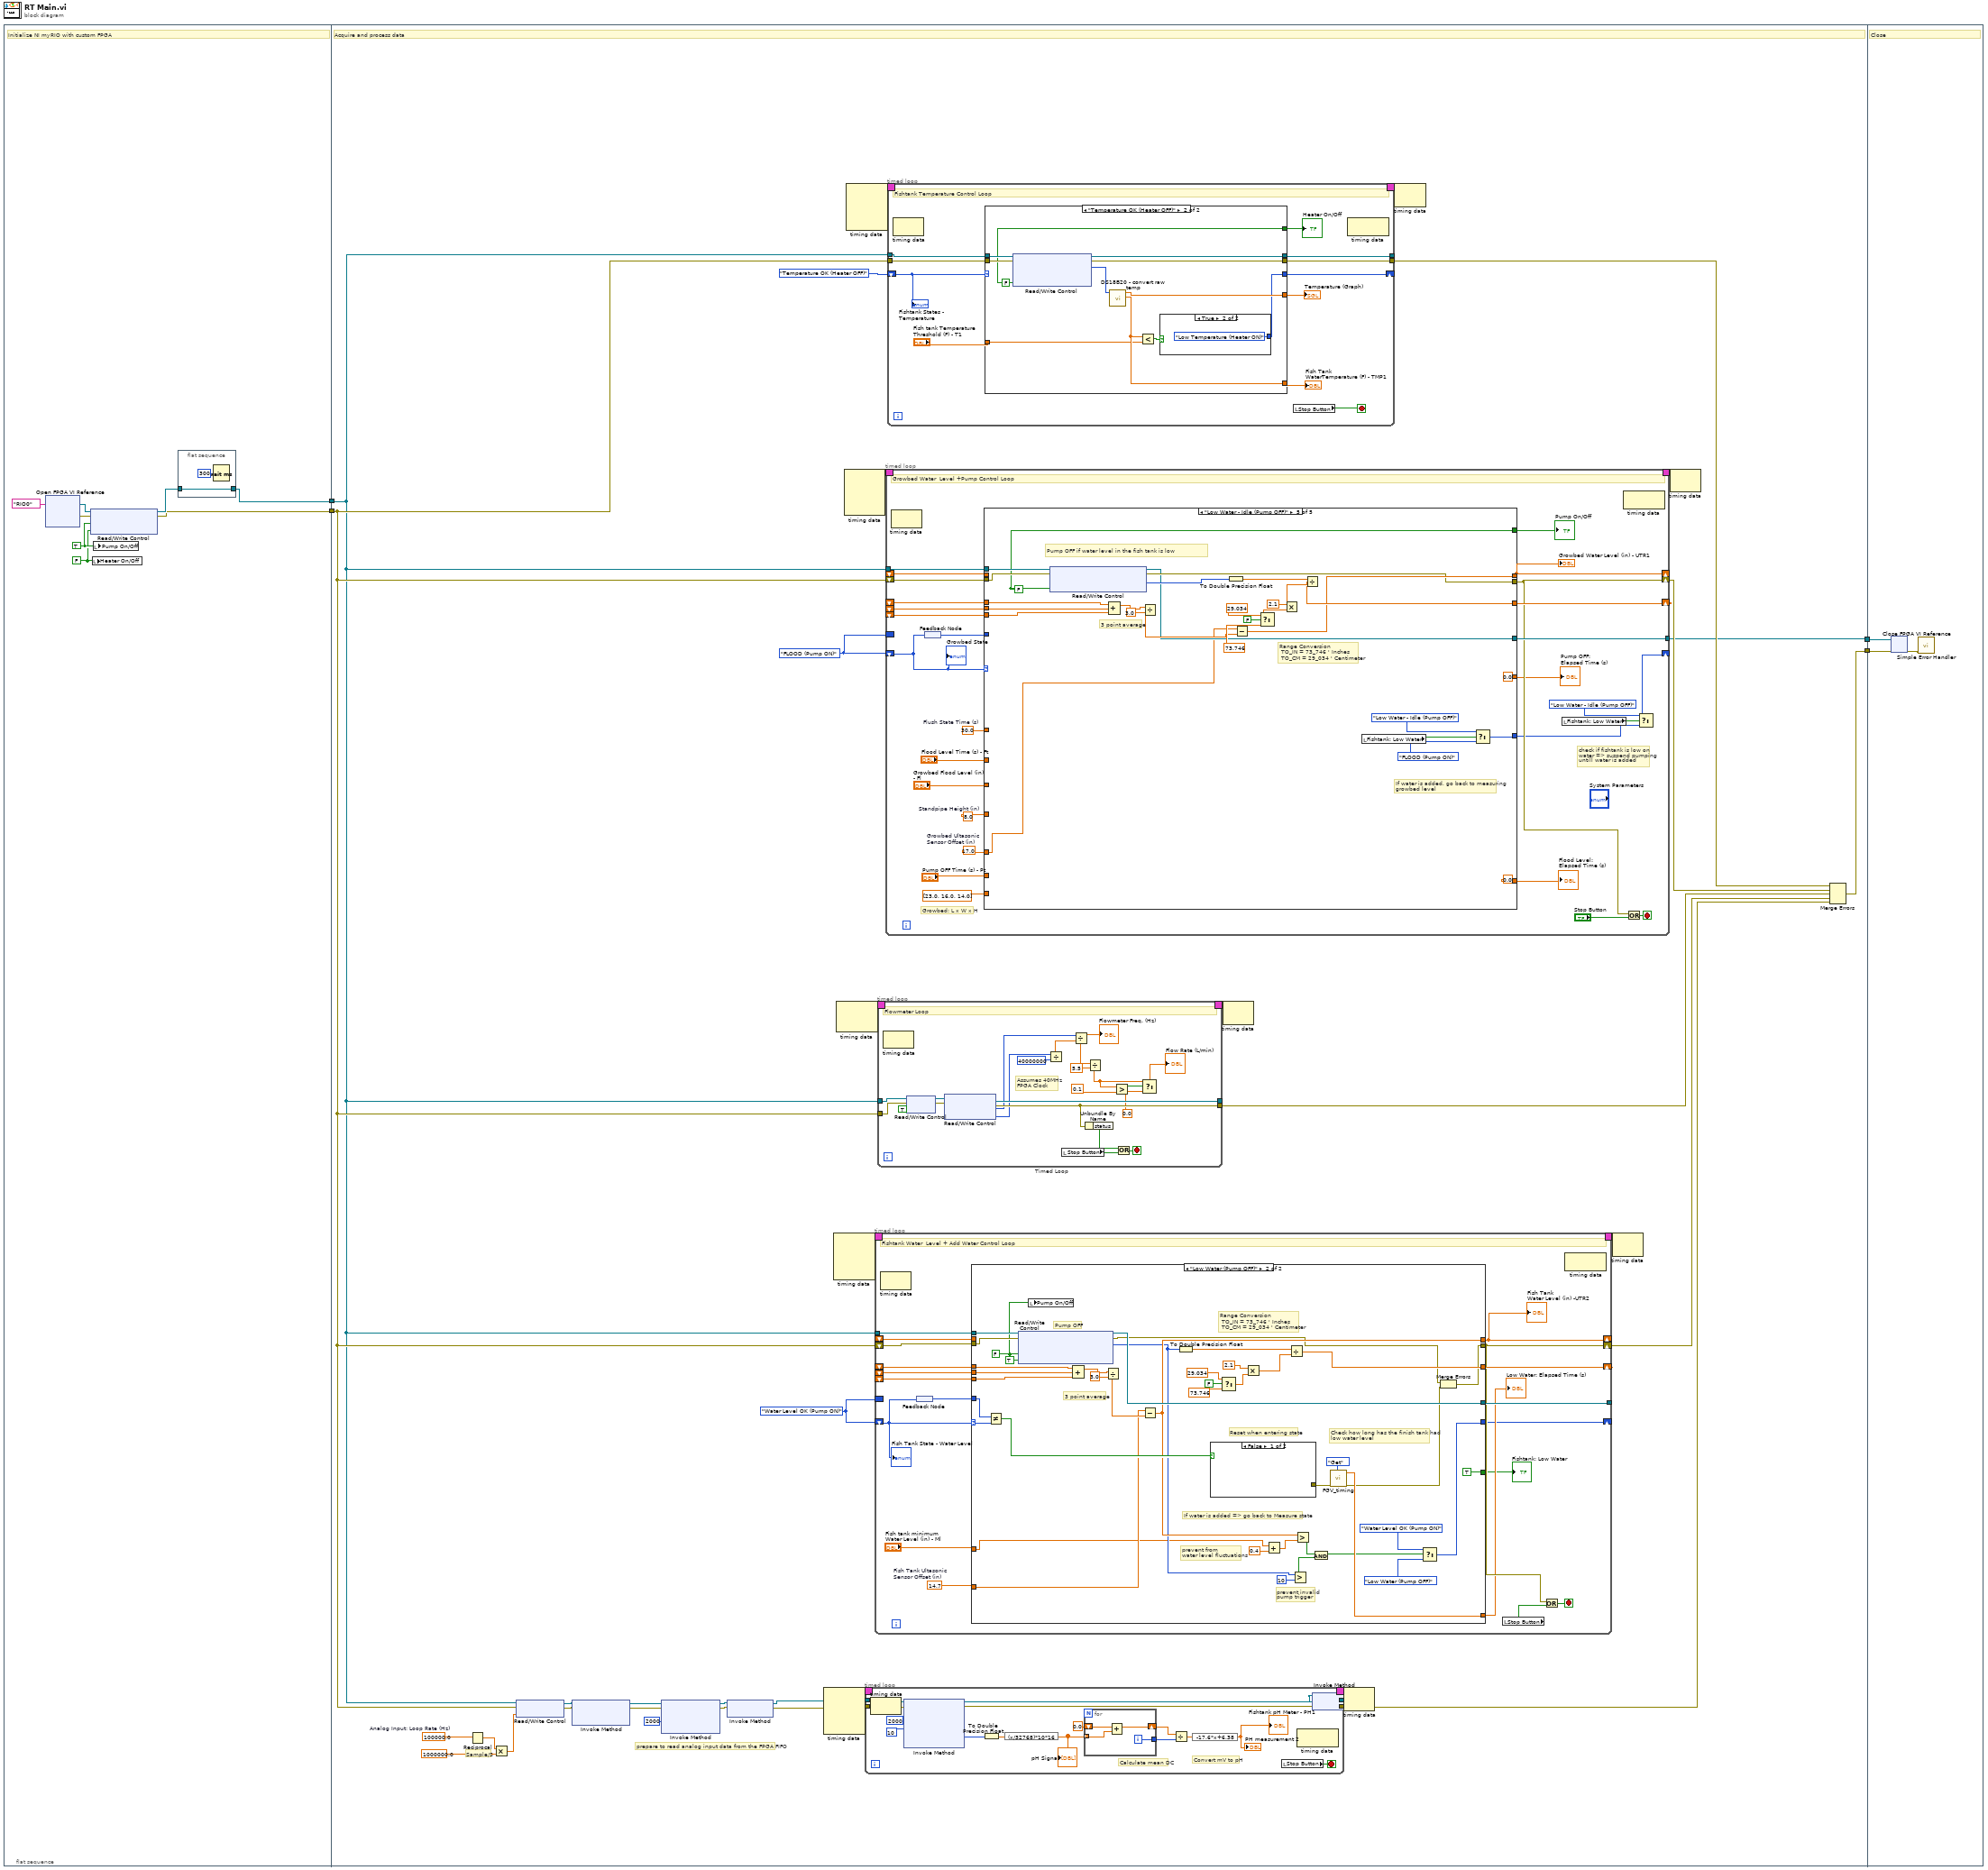
[diagram p0: block diagram]
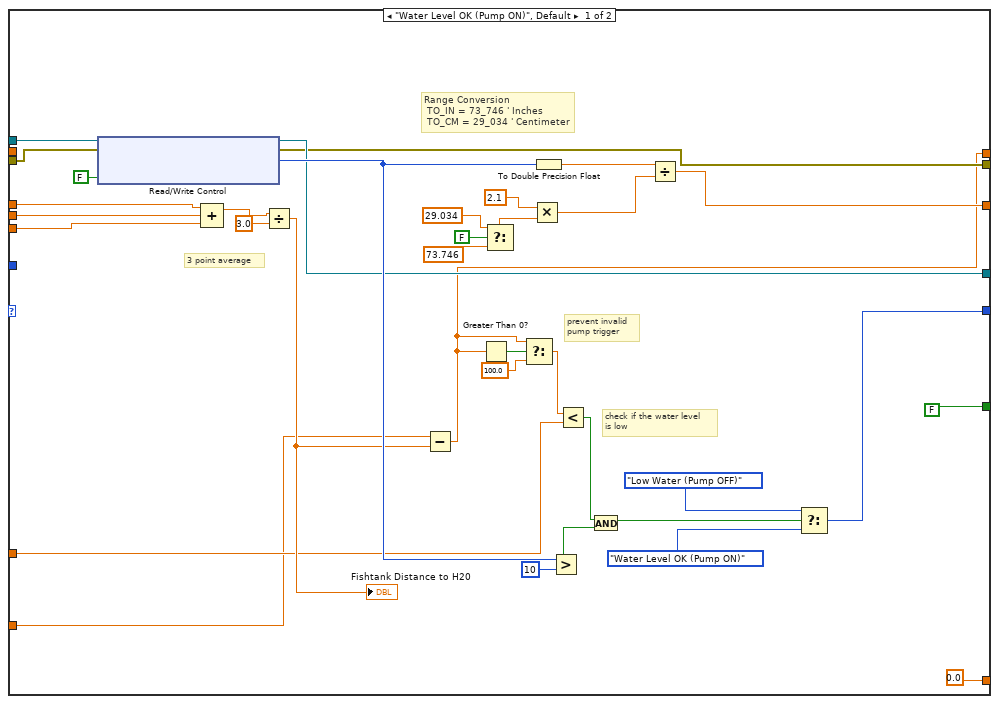
[diagram p2: hidden frame]
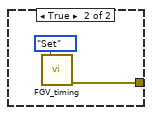
[diagram p3: hidden frame]
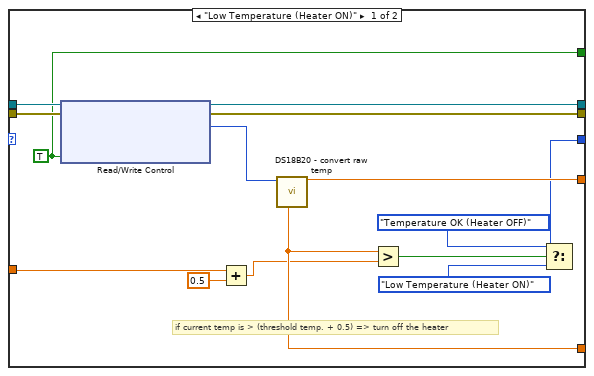
[diagram p4: hidden frame]
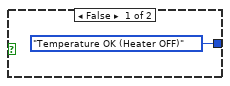
[diagram p5: hidden frame]
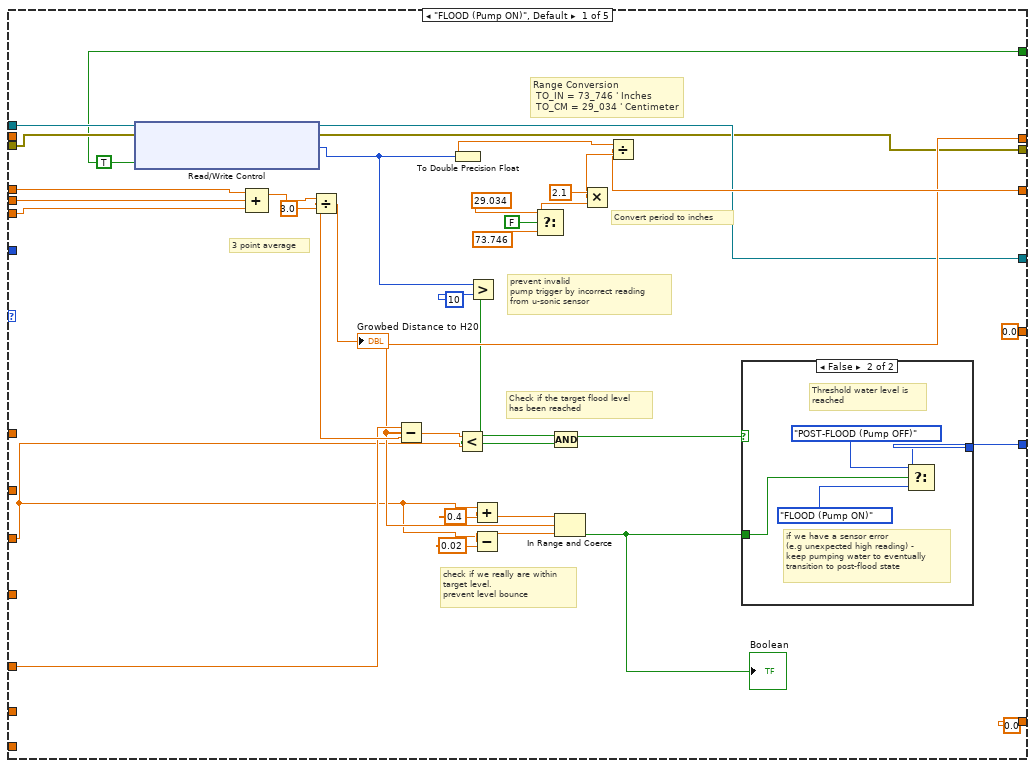
[diagram p6: hidden frame]
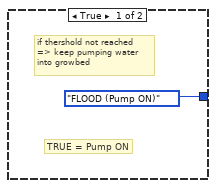
[diagram p7: hidden frame]
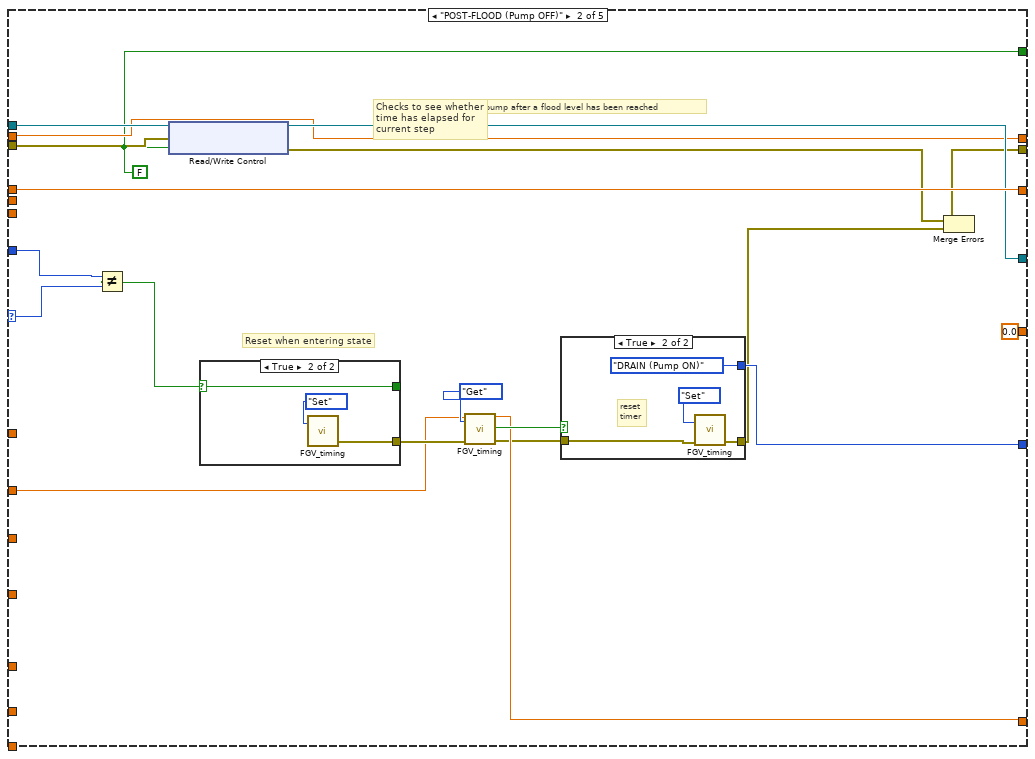
[diagram p8: hidden frame]
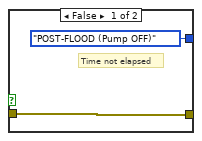
[diagram p10: hidden frame]
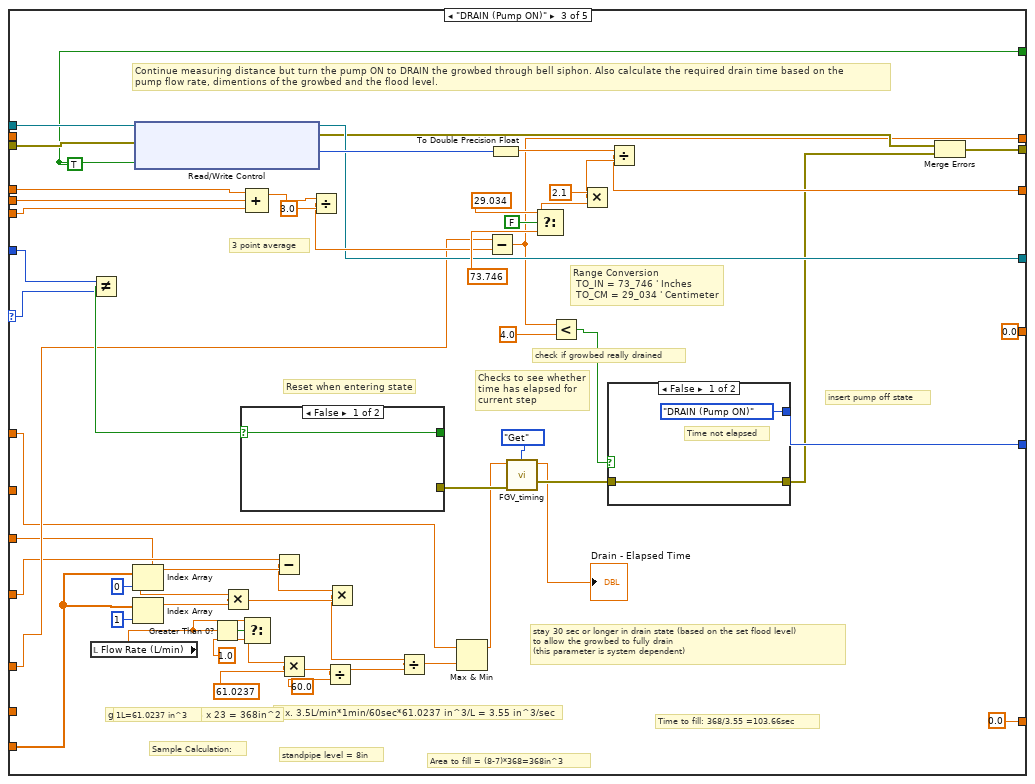
[diagram p11: hidden frame]
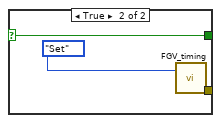
[diagram p12: hidden frame]
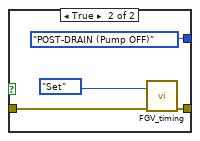
[diagram p13: hidden frame]
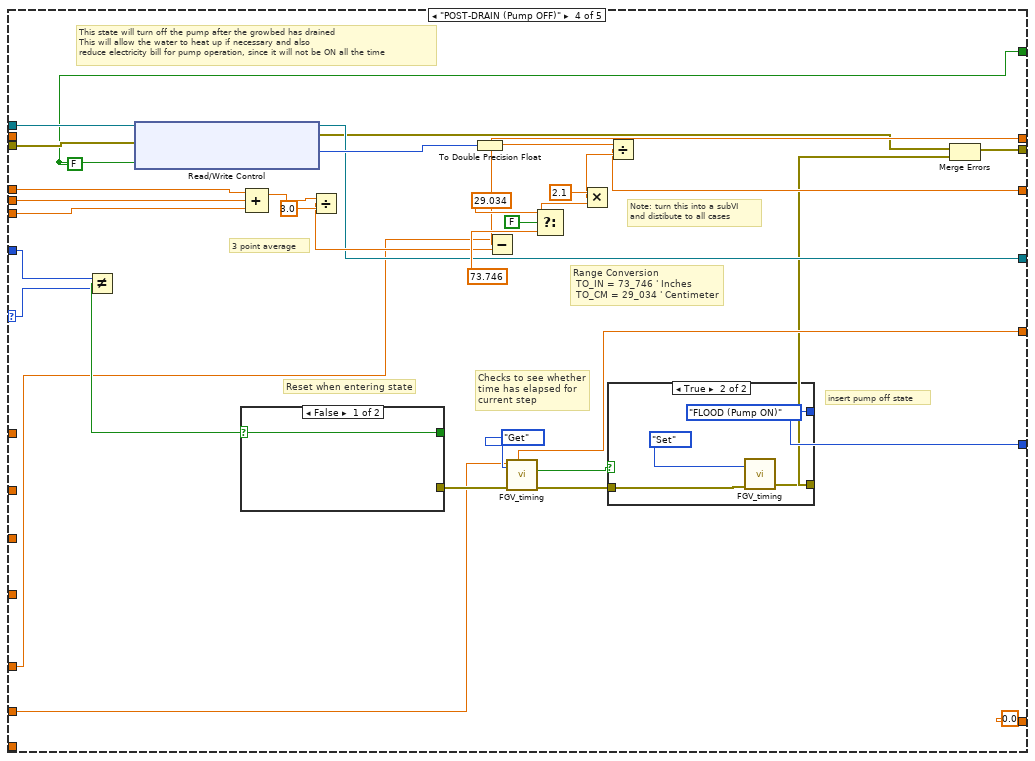
[diagram p14: hidden frame]
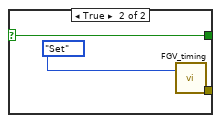
[diagram p15: hidden frame]
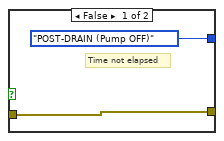
[diagram p16: hidden frame]
diagram:
  n1 = flat-sequence {
    tunnel: [w12] -> w4
    tunnel: [w7] -> w2
    tunnel: w4 -> [w16]
    tunnel: [w21] -> w3
    tunnel: w2 -> [w26]
    tunnel: [w15] -> w1
    tunnel: w3 -> [w487]
    tunnel: w1 -> [w488]
    frame #0 {
      w6 = FALSE ("Heater Control On/Off")
      w8 = TRUE ("Pump On/Off")
      # "Initialize NI myRIO with custom FPGA"
      n2 = xnode "Open FPGA VI Reference"("resource name"=tag "RIO0") -> ("FPGA VI Reference Out"=w11:refnum<k20>, "error out"=w9:errorcluster)  [unwired: 1 in]
      n3 = xnode "Read/Write Control"("FPGA VI Reference In"=w11, "error in"=w9, "Pump Control On/Off"=w8, "Heater Control On/Off"=w6) -> ("FPGA VI Reference Out"=w10:refnum<k20>, "error out"=w7:errorcluster)
      n4 = local write "Heater On/Off"(w6) -> ()
      n5 = local write "Pump On/Off"(w8) -> ()
      n6 = flat-sequence {
        tunnel: w10 -> [w14]
        tunnel: [w14] -> w12
        frame #0 {
          n7 = Wait (ms)(milliseconds to wait=u32 300) -> ()  [unwired: 1 out]
        }
      }
    }
    frame #1 {
      w17 = 100000.0  # Analog Input: Loop Rate (Hz)
      w40 = fishtank_level_states."Water Level OK (Pump ON)"
      w44 = growbed_states."FLOOD (Pump ON)"
      # "prepare to read analog input data from the FPGA FIFO"
      # "Sample/S"
      # "Acquire and process data"
      n8 = Reciprocal(x=w17) -> (1/x=w36:dbl)
      n9 = Multiply(x=w36, y=1000000.0) -> (x*y=w35:dbl)
      n10 = xnode "Read/Write Control"("FPGA VI Reference In"=w16, "error in"=w26, "Loop Rate (uS)"=w35) -> ("FPGA VI Reference Out"=w37:refnum<k20>, "error out"=w38:errorcluster)
      n11 = xnode "Invoke Method"("FPGA VI Reference In"=w37, "error in"=w38) -> ("FPGA VI Reference Out"=w34:refnum<k20>, "error out"=w33:errorcluster)  [unwired: 1 in]
      n12 = xnode "Invoke Method"("FPGA VI Reference In"=w34, "error in"=w33, "Requested Depth"=u32 2000) -> ("FPGA VI Reference Out"=w32:refnum<k20>, "error out"=w31:errorcluster)  [unwired: 1 out]
      n13 = xnode "Invoke Method"("FPGA VI Reference In"=w32, "error in"=w31) -> ("FPGA VI Reference Out"=w30:refnum<k20>, "error out"=w29:errorcluster)
      n14 = node-c288() -> (w25:T4)  [unwired: 4 in]
      n15 = node-c288() -> (w42:T4)  [unwired: 4 in]
      n16 = node-c288() -> (w48:T4)  [unwired: 2 out]
      n17 = node-c288() -> (w50:T4)  [unwired: 4 in]
      n18 = node-c288() -> (w46:T4)  [unwired: 4 in]
      n19 = timed-loop {
        tunnel: w30 -> [w65]
        tunnel: w29 -> [w64]
        tunnel: [w63] -> w28
        tunnel: [w62] -> w20
        timing: w25 -> [_]
        timing-out: [_] -> w24
        stop <- w51 stop-if-true
        # "Convert mV to pH"
        # "Calculate mean DC"
        n20 = node-c288() -> ()  [unwired: 1 in, 1 out]
        n21 = xnode "Invoke Method"("FPGA VI Reference In"=w65, "error in"=w64, "Number of Elements"=u32 2000, "Timeout (ms)"=10) -> ("FPGA VI Reference Out"=w63:refnum<k20>, "error out"=w62:errorcluster, "Data"=w59:i16[])  [unwired: 1 out]
        n22 = To Double Precision Float(number=w59) -> (double precision float=w58:dbl[])
        n23 = expression code="(x/32768)*10*16"(w58) -> (w54:dbl[])
        "pH Signal" <- w54
        n24 = for {
          shift-right: [w71] -> w56
          shift-left: 0.0 -> [w69]
          tunnel: [w70] -> w55
          tunnel: w54 -> [w68] mode=indexing
          i -> [w70]
          n25 = Add(x=w69, y=w68) -> (x+y=w71:dbl)
        }
        n26 = Divide(x=w56, y=w55) -> (x/y=w53:dbl)
        n27 = expression code="-17.6*x+6.38"(w53) -> (→"PH measurement 2" →"Fishtank pH Meter - PH1":dbl)
        n28 = local read "Stop Button"() -> (w51:bool)
        n29 = node-c288() -> ()  [unwired: 1 in, 1 out]
      }
      n30 = timed-loop {
        tunnel: w16 -> [w85]
        shift-right: [w86] -> w19
        shift-left: w26 -> [w92]
        timing: w42 -> [_]
        timing-out: [_] -> w41
        shift-right: [w91] -> _
        shift-left: _ -> [w90]
        shift-left: _ -> [w89]
        shift-left: _ -> [w88]
        tunnel: [w87] -> _
        shift-right: [w81] -> _
        shift-left: _ -> [w84]
        border: w40 -> [_]
        shift-right: [w78] -> _
        shift-left: w40 -> [w80]
        stop <- w76 stop-if-true
        w74 = 14.7  # Fish Tank Ultasonic Sensor Offset (in)
        # "Fishtank Water  Level + Add Water Control Loop"
        n31 = node-c288() -> ()  [unwired: 1 in, 1 out]
        n32 = feedback-in #1(w80) -> ()
        n33 = feedback #1() -> (w82:T2)
        n34 = case shown="\"Low Water (Pump OFF)\"" w80 {
          selector: w80 -> [_ w149]
          tunnel: w92 -> [w116 w162]
          tunnel: [w115 w161] -> w91
          tunnel: w90 -> [w114 w160]
          tunnel: w89 -> [w113 w159]
          tunnel: w88 -> [w112 w158]
          tunnel: [w104 w154] -> w87
          tunnel: [w103 w129] -> w86
          tunnel: w85 -> [w110 w157]
          tunnel: "Fish tank minimum\nWater Level (in) - Ml" -> [w108 w134]
          tunnel: [w96 w138] -> w81
          tunnel: w84 -> [_ _]
          tunnel: [0.0 ("Elapsed Time") w146] -> w83
          tunnel: w82 -> [_ w150]
          tunnel: w74 -> [w106 w147]
          tunnel: [w99 w139] -> w78
          tunnel: [FALSE ("s") TRUE ("s")] -> w77
          frame "Water Level OK (Pump ON)", Default {
            # "check if the water level\nis low"
            # "prevent invalid\npump trigger"
            # "Range Conversion\n TO_IN = 73_746 ' Inches \n TO_CM = 29_034 ' Centimeter"
            # "3 point average"
            n35 = xnode "Read/Write Control"("FPGA VI Reference In"=w110, "error in"=w116, "Add Water Control On/Off"=FALSE) -> ("FPGA VI Reference Out"=w104:refnum<k20>, "error out"=w103:errorcluster, "Measured Period (usec) - Fishtank"=w119:u32)
            n36 = Compound Arithmetic op=ADD(w114, w113, w112) -> (w122:dbl)
            n37 = Divide(x=w122, y=3.0) -> (x/y=w111:dbl)
            "Fishtank Distance to H20" <- w111
            n38 = Subtract(x=w106, y=w111) -> (x-y=w96:dbl)
            n39 = Greater Than 0?(x=w96) -> (x > 0?=w97:bool)
            n40 = Select(t=29.034 ("x"), s=FALSE, f=73.746 ("x")) -> (s? t:f=w124:dbl)
            n41 = Select(t=w96, s=w97, f=100.0) -> (s? t:f=w94:dbl)
            n42 = Multiply(x=2.1, y=w124) -> (x*y=w123:dbl)
            n43 = To Double Precision Float(number=w119) -> (double precision float=w109:dbl)
            n44 = Greater?(x=w119, y=u32 10) -> (0:w117:bool)
            n45 = Less?(x=w94, y=w108) -> (x < y?=w120:bool)
            n46 = And(x=w120, y=w117) -> (x .and. y?=w102:bool)
            n47 = Divide(x=w109, y=w123) -> (x/y=w115:dbl)
            n48 = Select(t=fishtank_level_states."Low Water (Pump OFF)", s=w102, f=fishtank_level_states."Water Level OK (Pump ON)") -> (s? t:f=w99:T2)
          }
          frame "Low Water (Pump OFF)" {
            w135 = FALSE ("Pump Control On/Off")
            # "prevent from\nwater level fluctuations"
            # "If water is added => go back to Measure state"
            # "prevent invalid\npump trigger"
            # "Pump OFF"
            # "Reset when entering state"
            # "Check how long has the finish tank had\nlow water level"
            # "Range Conversion\n TO_IN = 73_746 ' Inches \n TO_CM = 29_034 ' Centimeter"
            # "3 point average"
            n49 = Not Equal?(x=w150, y=w149) -> (x != y?=w151:bool)
            n50 = xnode "Read/Write Control"("FPGA VI Reference In"=w157, "error in"=w162, "Pump Control On/Off"=w135, "Add Water Control On/Off"=TRUE) -> ("FPGA VI Reference Out"=w154:refnum<k20>, "error out"=w130:errorcluster, "Measured Period (usec) - Fishtank"=w137:u32)
            n51 = local write "Pump On/Off"(w135) -> ()
            n52 = Compound Arithmetic op=ADD(w160, w159, w158) -> (w164:dbl)
            n53 = Divide(x=w164, y=3.0) -> (x/y=w148:dbl)
            n54 = Subtract(x=w147, y=w148) -> (x-y=w138:dbl)
            n55 = To Double Precision Float(number=w137) -> (double precision float=w156:dbl)
            n56 = case shown="False" w151 {
              tunnel: [_ w170] -> w152
              frame False {
              }
              frame True {
                n57 = call "FGV_timing.vi"("Enum"=FGV_enum."Set") -> ("error out"=w170:errorcluster)  [unwired: 8 in, 2 out]
              }
            }
            n58 = Select(t=29.034 ("x"), s=FALSE, f=73.746 ("x")) -> (s? t:f=w166:dbl)
            n59 = Multiply(x=2.1, y=w166) -> (x*y=w165:dbl)
            n60 = Add(x=w134, y=0.4) -> (x+y=w132:dbl)
            n61 = Divide(x=w156, y=w165) -> (x/y=w161:dbl)
            n62 = Greater?(x=w137, y=u32 10) -> (0:w143:bool)
            n63 = Greater?(x=w138, y=w132) -> (0:w145:bool)
            n64 = And(x=w145, y=w143) -> (x .and. y?=w142:bool)
            n65 = call "FGV_timing.vi"("Enum"=FGV_enum."Get", "error in (no error)"=w152) -> ("error out"=w131:errorcluster, "Elapsed Time"=w146:dbl)  [unwired: 7 in, 1 out]
            n66 = Select(t=fishtank_level_states."Water Level OK (Pump ON)", s=w142, f=fishtank_level_states."Low Water (Pump OFF)") -> (s? t:f=w139:T2)
            n67 = Merge Errors(w130, w131) -> (w129:errorcluster)
          }
        }
        "Low Water: Elapsed Time (s)" <- w83
        "Fish Tank\nWater Level (in) -UTR2" <- w81
        "Fishtank: Low Water" <- w77
        n68 = local read "Stop Button"() -> (w75:bool)
        n69 = Or(x=w86, y=w75) -> (x .or. y?=w76:bool)
        n70 = node-c288() -> ()  [unwired: 1 in, 1 out]
        "Fish Tank State - Water Level" <- w80
      }
      n71 = timed-loop "Timed Loop" {
        tunnel: [w230] -> w18
        tunnel: [w231] -> _
        tunnel: w26 -> [w238]
        tunnel: w16 -> [w239]
        timing-out: [_] -> w47
        timing: w48 -> [_]
        stop <- w233 stop-if-true
        # "Assumes 40MHz FPGA Clock"
        # "Flowmeter Loop"
        n72 = node-c288() -> ()  [unwired: 2 out]
        n73 = xnode "Read/Write Control"("FPGA VI Reference In"=w239, "error in"=w238, "Sample"=TRUE) -> ("FPGA VI Reference Out"=w236:refnum<k20>, "error out"=w235:errorcluster)
        n74 = xnode "Read/Write Control"("FPGA VI Reference In"=w236, "error in"=w235) -> ("FPGA VI Reference Out"=w231:refnum<k20>, "error out"=w230:errorcluster, "Flowrate: Count"=w227:u32, "Flowrate: Period"=w228:u32)
        n75 = Divide(x=w228, y=40000000) -> (x/y=w232:dbl)
        n76 = local read "Stop Button"() -> (w224:bool)
        n77 = Divide(x=w227, y=w232) -> (x/y=w226:dbl)
        "Flowmeter Freq. (Hz)" <- w226
        n78 = Unbundle By Name(w230) -> ("status"=w234:bool)
        n79 = Divide(x=w226, y=5.5) -> (x/y=w219:dbl)
        n80 = Greater?(x=w219, y=0.1) -> (0:w222:bool)
        n81 = Or(x=w234, y=w224) -> (x .or. y?=w233:bool)
        n82 = Select(t=w219, s=w222, f=0.0) -> (s? t:f=→"Flow Rate (L/min)":dbl)
      }
      n83 = timed-loop {
        tunnel: w16 -> [w262]
        shift-right: [w263] -> w22
        shift-left: w26 -> [w269]
        timing: w50 -> [_]
        timing-out: [_] -> w49
        shift-right: [w268] -> _
        shift-left: _ -> [w267]
        shift-left: _ -> [w266]
        shift-left: _ -> [w265]
        tunnel: [w264] -> w15
        shift-right: [w260] -> _
        shift-left: _ -> [w244]
        shift-right: [w250] -> _
        shift-left: w44 -> [w258]
        border: w44 -> [_]
        stop <- w270 stop-if-true
        w248 = 8.0  # Standpipe Height (in)
        w254 = 30.0  # Flush State Time (s)
        w256 = 17.0  # Growbed Ultasonic Sensor Offset (in)
        # "Growbed: L x W x H"
        # "check if fishtank is low on \nwater => suspend pumping\nuntill water is added"
        # "Growbed Water  Level +Pump Control Loop"
        n84 = node-c288() -> ()  [unwired: 1 in, 1 out]
        n85 = feedback-in #2(w258) -> ()
        n86 = feedback #2() -> (w257:T3)
        n87 = case shown="\"Low Water - Idle (Pump OFF)\"" w258 {
          selector: w258 -> [_ w324 w375 w418 _]
          tunnel: w269 -> [w296 w317 w390 w435 w473]
          tunnel: [w295 w330 w389 w434 w472] -> w268
          tunnel: w267 -> [w294 w330 w388 w433 w471]
          tunnel: w266 -> [w293 _ w387 w432 w470]
          tunnel: w265 -> [w292 _ w386 w431 w469]
          tunnel: [w276 w319 w382 w426 w463] -> w264
          tunnel: [w275 w312 w345 w409 w464] -> w263
          tunnel: w262 -> [w290 w331 w384 w429 w467]
          tunnel: [w289 w329 w374 w417 w457] -> w251
          tunnel: "Growbed Flood Level (in) - Fl" -> [w274 _ w359 _ _]
          tunnel: [w281 w318 w344 w427 w465] -> w260
          tunnel: w244 -> [_ w318 _ _ _]
          tunnel: "Flood Level Time (s) - Ft" -> [_ w321 _ _ _]
          tunnel: [0.0 ("Elapsed Time") w326 0.0 ("Elapsed Time") 0.0 ("Elapsed Time") 0.0 ("Elapsed Time")] -> w245
          tunnel: w257 -> [_ w322 w376 w419 _]
          tunnel: w256 -> [w286 _ w372 w415 w460]
          tunnel: "Pump OFF Time (s) - Pt" -> [_ _ _ w413 _]
          tunnel: w254 -> [_ _ w355 _ _]
          tunnel: dbl[] [23.0, 16.0, 14.0] -> [_ _ w363 _ _]
          tunnel: w248 -> [_ _ w360 _ _]
          tunnel: [0.0 ("Elapsed Time") 0.0 ("Elapsed Time") 0.0 ("Elapsed Time") w414 0.0 ("Elapsed Time")] -> w247
          tunnel: [w277 w316 w348 w412 w454] -> w246
          frame "FLOOD (Pump ON)", Default {
            w277 = TRUE ("Pump Control On/Off")
            # "Convert period to inches"
            # "Check if the target flood level\nhas been reached"
            # "check if we really are within\ntarget level.\nprevent level bounce"
            # "prevent invalid\npump trigger by incorrect reading\nfrom u-sonic sensor"
            # "Range Conversion\n TO_IN = 73_746 ' Inches \n TO_CM = 29_034 ' Centimeter"
            # "3 point average"
            n88 = xnode "Read/Write Control"("FPGA VI Reference In"=w290, "error in"=w296, "Pump Control On/Off"=w277) -> ("FPGA VI Reference Out"=w276:refnum<k20>, "error out"=w275:errorcluster, "Measured Period (usec) - Growbed"=w298:u32)
            n89 = Compound Arithmetic op=ADD(w294, w293, w292) -> (w301:dbl)
            n90 = Divide(x=w301, y=3.0) -> (x/y=w291:dbl)
            "Growbed Distance to H20" <- w291
            n91 = Subtract(x=w286, y=w291) -> (x-y=w281:dbl)
            n92 = To Double Precision Float(number=w298) -> (double precision float=w288:dbl)
            n93 = Less?(x=w281, y=w274) -> (x < y?=w272:bool)
            n94 = Greater?(x=w298, y=u32 10) -> (0:w273:bool)
            n95 = Add(x=w274, y=0.4) -> (x+y=w282:dbl)
            n96 = Subtract(x=w274, y=0.02) -> (x-y=w278:dbl)
            n97 = Select(t=29.034 ("x"), s=FALSE, f=73.746 ("x")) -> (s? t:f=w303:dbl)
            n98 = Compound Arithmetic op=AND(w273, w272) -> (w299:bool)
            n99 = In Range and Coerce(upper limit=w282, x=w281, lower limit=w278) -> (In Range?=w280:bool)  [unwired: 1 out]
            "Boolean" <- w280
            n100 = Multiply(x=2.1, y=w303) -> (x*y=w302:dbl)
            n101 = Divide(x=w288, y=w302) -> (x/y=w295:dbl)
            n102 = case shown="False" w299 {
              tunnel: [growbed_states."FLOOD (Pump ON)" w308] -> w289
              tunnel: w280 -> [_ w311]
              frame True {
                # "TRUE = Pump ON"
                # "if thershold not reached\n=> keep pumping water\ninto growbed"
              }
              frame False {
                # "if we have a sensor error \n(e.g unexpected high reading) - \nkeep pumping water to eventually\ntransition to post-flood state"
                # "Threshold water level is\nreached"
                n103 = Select(t=growbed_states."POST-FLOOD (Pump OFF)", s=w311, f=growbed_states."FLOOD (Pump ON)") -> (s? t:f=w308:T3)
              }
            }
          }
          frame "POST-FLOOD (Pump OFF)" {
            w316 = FALSE ("Pump Control On/Off")
            # "This state will pause the pump after a flood level has been reached"
            # "Reset when entering state"
            # "Checks to see whether\ntime has elapsed for \ncurrent step"
            n104 = Not Equal?(x=w322, y=w324) -> (x != y?=w323:bool)
            n105 = xnode "Read/Write Control"("FPGA VI Reference In"=w331, "error in"=w317, "Pump Control On/Off"=w316) -> ("FPGA VI Reference Out"=w319:refnum<k20>, "error out"=w313:errorcluster)
            n106 = case shown="True" w323 {
              selector: w323 -> [w332 w333]
              tunnel: [_ w334] -> w325
              tunnel: [w332 w333] -> _
              frame False {
              }
              frame True {
                n107 = call "FGV_timing.vi"("Enum"=FGV_enum."Set") -> ("error out"=w334:errorcluster)  [unwired: 8 in, 2 out]
              }
            }
            n108 = call "FGV_timing.vi"("Enum"=FGV_enum."Get", "error in (no error)"=w325, "Target time"=w321) -> ("error out"=w315:errorcluster, "Elapsed?"=w327:bool, "Elapsed Time"=w326:dbl)  [unwired: 6 in]
            n109 = case shown="True" w327 {
              tunnel: w315 -> [w337 w338]
              tunnel: [w337 w341] -> w314
              tunnel: [growbed_states."POST-FLOOD (Pump OFF)" growbed_states."DRAIN (Pump ON)"] -> w329
              frame False {
                # "Time not elapsed"
              }
              frame True {
                # "reset\ntimer"
                n110 = call "FGV_timing.vi"("Enum"=FGV_enum."Set", "error in (no error)"=w338) -> ("error out"=w341:errorcluster)  [unwired: 7 in, 2 out]
              }
            }
            n111 = Merge Errors(w313, w314) -> (w312:errorcluster)
          }
          frame "DRAIN (Pump ON)" {
            w348 = TRUE ("Pump Control On/Off")
            # "check if growbed really drained"
            # "Sample Calculation:"
            # "Time to fill: 368/3.55 =103.66sec"
            # "Area to fill = (8-7)*368=368in^3"
            # "standpipe level = 8in"
            # "growbed area =  16 x 23 = 368in^2"
            # "E.x. 3.5L/min*1min/60sec*61.0237 in^3/L = 3.55 in^3/sec"
            # "1L=61.0237 in^3"
            # "insert pump off state"
            # "Continue measuring distance but turn the pump ON to DRAIN the growbed through bell siphon. Also calculate the required drain time based on the \npump flow rate, dimentions of the growbed and the flood level."
            # "stay 30 sec or longer in drain state (based on the set flood level)\nto allow the growbed to fully drain\n(this parameter is system dependent)"
            # "Reset when entering state"
            # "Checks to see whether\ntime has elapsed for \ncurrent step"
            # "Range Conversion\n TO_IN = 73_746 ' Inches \n TO_CM = 29_034 ' Centimeter"
            # "3 point average"
            n112 = Not Equal?(x=w376, y=w375) -> (x != y?=w377:bool)
            n113 = local read "Flow Rate (L/min)"() -> (w352:dbl)
            n114 = Index Array(array=w363, index=0) -> (element=w362:dbl)
            n115 = Index Array(array=w363, index=1) -> (element=w361:dbl)
            n116 = xnode "Read/Write Control"("FPGA VI Reference In"=w384, "error in"=w390, "Pump Control On/Off"=w348) -> ("FPGA VI Reference Out"=w382:refnum<k20>, "error out"=w347:errorcluster, "Measured Period (usec) - Growbed"=w391:u32)
            n117 = Greater Than 0?(x=w352) -> (x > 0?=w353:bool)
            n118 = Multiply(x=w362, y=w361) -> (x*y=w357:dbl)
            n119 = case shown="False" w377 {
              selector: w377 -> [w399 w400]
              tunnel: [_ w401] -> w378
              tunnel: [w399 w400] -> _
              frame False {
              }
              frame True {
                n120 = call "FGV_timing.vi"("Enum"=FGV_enum."Set") -> ("error out"=w401:errorcluster)  [unwired: 8 in, 2 out]
              }
            }
            n121 = Select(t=w352, s=w353, f=1.0) -> (s? t:f=w350:dbl)
            n122 = Compound Arithmetic op=ADD(w388, w387, w386) -> (w393:dbl)
            n123 = Subtract(x=w360, y=w359) -> (x-y=w358:dbl)
            n124 = Multiply(x=w350, y=61.0237) -> (x*y=w369:dbl)
            n125 = Divide(x=w393, y=3.0) -> (x/y=w385:dbl)
            n126 = Divide(x=w369, y=60.0) -> (x/y=w367:dbl)
            n127 = Multiply(x=w358, y=w357) -> (x*y=w356:dbl)
            n128 = Divide(x=w356, y=w367) -> (x/y=w366:dbl)
            n129 = Max & Min(x=w355, y=w366) -> (max(x,y)=w354:dbl)  [unwired: 1 out]
            n130 = Subtract(x=w372, y=w385) -> (x-y=w344:dbl)
            n131 = To Double Precision Float(number=w391) -> (double precision float=w383:dbl)
            n132 = call "FGV_timing.vi"("Enum"=FGV_enum."Get", "error in (no error)"=w378, "Target time"=w354) -> ("error out"=w379:errorcluster, "Elapsed Time"=→"Drain - Elapsed Time":dbl)  [unwired: 6 in, 1 out]
            n133 = Select(t=29.034 ("x"), s=FALSE, f=73.746 ("x")) -> (s? t:f=w395:dbl)
            n134 = Less?(x=w344, y=4.0) -> (x < y?=w342:bool)
            n135 = Multiply(x=2.1, y=w395) -> (x*y=w394:dbl)
            n136 = case shown="False" w342 {
              tunnel: w379 -> [w404 w408]
              tunnel: [w404 w407] -> w346
              tunnel: [growbed_states."DRAIN (Pump ON)" growbed_states."POST-DRAIN (Pump OFF)"] -> w374
              frame False {
                # "Time not elapsed"
              }
              frame True {
                n137 = call "FGV_timing.vi"("Enum"=FGV_enum."Set", "error in (no error)"=w408) -> ("error out"=w407:errorcluster)  [unwired: 7 in, 2 out]
              }
            }
            n138 = Divide(x=w383, y=w394) -> (x/y=w389:dbl)
            n139 = Merge Errors(w347, w346) -> (w345:errorcluster)
          }
          frame "POST-DRAIN (Pump OFF)" {
            w412 = FALSE ("Pump Control On/Off")
            # "Note: turn this into a subVI\nand distibute to all cases"
            # "insert pump off state"
            # "This state will turn off the pump after the growbed has drained\nThis will allow the water to heat up if necessary and also  \nreduce electricity bill for pump operation, since it will not be ON all the time"
            # "Reset when entering state"
            # "Checks to see whether\ntime has elapsed for \ncurrent step"
            # "Range Conversion\n TO_IN = 73_746 ' Inches \n TO_CM = 29_034 ' Centimeter"
            # "3 point average"
            n140 = Not Equal?(x=w419, y=w418) -> (x != y?=w420:bool)
            n141 = xnode "Read/Write Control"("FPGA VI Reference In"=w429, "error in"=w435, "Pump Control On/Off"=w412) -> ("FPGA VI Reference Out"=w426:refnum<k20>, "error out"=w410:errorcluster, "Measured Period (usec) - Growbed"=w436:u32)
            n142 = case shown="False" w420 {
              selector: w420 -> [w444 w445]
              tunnel: [_ w446] -> w421
              tunnel: [w444 w445] -> _
              frame False {
              }
              frame True {
                n143 = call "FGV_timing.vi"("Enum"=FGV_enum."Set") -> ("error out"=w446:errorcluster)  [unwired: 8 in, 2 out]
              }
            }
            n144 = Compound Arithmetic op=ADD(w433, w432, w431) -> (w438:dbl)
            n145 = Divide(x=w438, y=3.0) -> (x/y=w430:dbl)
            n146 = To Double Precision Float(number=w436) -> (double precision float=w428:dbl)
            n147 = Subtract(x=w415, y=w430) -> (x-y=w427:dbl)
            n148 = call "FGV_timing.vi"("Enum"=FGV_enum."Get", "error in (no error)"=w421, "Target time"=w413) -> ("error out"=w422:errorcluster, "Elapsed?"=w423:bool, "Elapsed Time"=w414:dbl)  [unwired: 6 in]
            n149 = Select(t=29.034 ("x"), s=FALSE, f=73.746 ("x")) -> (s? t:f=w440:dbl)
            n150 = Multiply(x=2.1, y=w440) -> (x*y=w439:dbl)
            n151 = Divide(x=w428, y=w439) -> (x/y=w434:dbl)
            n152 = case shown="True" w423 {
              tunnel: w422 -> [w449 w453]
              tunnel: [w449 w452] -> w411
              tunnel: [growbed_states."POST-DRAIN (Pump OFF)" growbed_states."FLOOD (Pump ON)"] -> w417
              frame False {
                # "Time not elapsed"
              }
              frame True {
                n153 = call "FGV_timing.vi"("Enum"=FGV_enum."Set", "error in (no error)"=w453) -> ("error out"=w452:errorcluster)  [unwired: 7 in, 2 out]
              }
            }
            n154 = Merge Errors(w410, w411) -> (w409:errorcluster)
          }
          frame "Low Water - Idle (Pump OFF)" {
            w454 = FALSE ("Pump Control On/Off")
            # "If water is added, go back to measuring\ngrowbed level"
            # "Pump OFF if water level in the fish tank is low"
            # "Range Conversion\n TO_IN = 73_746 ' Inches \n TO_CM = 29_034 ' Centimeter"
            # "3 point average"
            n155 = xnode "Read/Write Control"("FPGA VI Reference In"=w467, "error in"=w473, "Pump Control On/Off"=w454) -> ("FPGA VI Reference Out"=w463:refnum<k20>, "error out"=w464:errorcluster, "Measured Period (usec) - Growbed"=w474:u32)
            n156 = Compound Arithmetic op=ADD(w471, w470, w469) -> (w476:dbl)
            n157 = Divide(x=w476, y=3.0) -> (x/y=w468:dbl)
            n158 = To Double Precision Float(number=w474) -> (double precision float=w466:dbl)
            n159 = Subtract(x=w460, y=w468) -> (x-y=w465:dbl)
            n160 = Select(t=29.034 ("x"), s=FALSE, f=73.746 ("x")) -> (s? t:f=w478:dbl)
            n161 = Multiply(x=2.1, y=w478) -> (x*y=w477:dbl)
            n162 = Divide(x=w466, y=w477) -> (x/y=w472:dbl)
            n163 = local read "Fishtank: Low Water"() -> (w456:bool)
            n164 = Select(t=growbed_states."Low Water - Idle (Pump OFF)", s=w456, f=growbed_states."FLOOD (Pump ON)") -> (s? t:f=w457:T3)
          }
        }
        "Growbed Water Level (in) - UTR1" <- w260
        "Flood Level: \nElapsed Time (s)" <- w245
        "Pump OFF:\nElapsed Time (s)" <- w247
        "Pump On/Off" <- w246
        n165 = local read "Fishtank: Low Water"() -> (w253:bool)
        n166 = node-c288() -> ()  [unwired: 1 in, 1 out]
        n167 = Or(x=w263, y="Stop Button") -> (x .or. y?=w270:bool)
        n168 = Select(t=growbed_states."Low Water - Idle (Pump OFF)", s=w253, f=w251) -> (s? t:f=w250:T3)
        "Growbed State" <- w258
      }
      n169 = timed-loop {
        timing: w46 -> [_]
        timing-out: [_] -> w45
        tunnel: w16 -> [w186]
        tunnel: w26 -> [w185]
        tunnel: [w184] -> _
        tunnel: [w183] -> w23
        shift-right: [w178] -> _
        shift-left: fishtank_states."Temperature OK (Heater OFF)" -> [w181]
        stop <- w182 stop-if-true
        # "Fishtank Temperature Control Loop"
        n170 = node-c288() -> ()  [unwired: 1 in, 1 out]
        n171 = case shown="\"Temperature OK (Heater OFF)\"" w181 {
          tunnel: w186 -> [w200 w211]
          tunnel: w185 -> [w199 w210]
          tunnel: [w198 w209] -> w184
          tunnel: [w197 w208] -> w183
          tunnel: [w188 w205] -> w180
          tunnel: [w196 w207] -> w179
          tunnel: [w190 w203] -> w178
          tunnel: "Fish tank Temperature\nThreshold (F) - T1" -> [w195 w204]
          tunnel: [w189 w202] -> w176
          frame "Low Temperature (Heater ON)" {
            w189 = TRUE ("Heater Control On/Off")
            # "if current temp is > (threshold temp. + 0.5) => turn off the heater"
            n172 = xnode "Read/Write Control"("FPGA VI Reference In"=w200, "error in"=w199, "Heater Control On/Off"=w189) -> ("FPGA VI Reference Out"=w198:refnum<k20>, "error out"=w197:errorcluster, "FishtankTemperature (raw)"=w201:u16)  [unwired: 1 out]
            n173 = Add(x=w195, y=0.5) -> (x+y=w187:dbl)
            n174 = call "DS18B20 - convert raw temp.vi"("Raw Temp"=w201) -> ("Temp (F)"=w188:sgl, "Temp (C)"=w196:sgl)  [unwired: 9 in]
            n175 = Greater?(x=w188, y=w187) -> (0:w193:bool)
            n176 = Select(t=fishtank_states."Temperature OK (Heater OFF)", s=w193, f=fishtank_states."Low Temperature (Heater ON)") -> (s? t:f=w190:T1)
          }
          frame "Temperature OK (Heater OFF)" {
            w202 = FALSE ("Heater Control On/Off")
            n177 = xnode "Read/Write Control"("FPGA VI Reference In"=w211, "error in"=w210, "Heater Control On/Off"=w202) -> ("FPGA VI Reference Out"=w209:refnum<k20>, "error out"=w208:errorcluster, "FishtankTemperature (raw)"=w212:u16)  [unwired: 1 out]
            n178 = call "DS18B20 - convert raw temp.vi"("Raw Temp"=w212) -> ("Temp (F)"=w205:sgl, "Temp (C)"=w207:sgl)  [unwired: 9 in]
            n179 = Less?(x=w205, y=w204) -> (x < y?=w206:bool)
            n180 = case shown="True" w206 {
              tunnel: [fishtank_states."Temperature OK (Heater OFF)" fishtank_states."Low Temperature (Heater ON)"] -> w203
              frame False {
              }
              frame True {
              }
            }
          }
        }
        "Temperature (Graph)" <- w179
        "Fish Tank \nWaterTemperature (F) - TMP1" <- w180
        "Heater On/Off" <- w176
        n181 = local read "Stop Button"() -> (w182:bool)
        n182 = node-c288() -> ()  [unwired: 1 in, 1 out]
        "Fishtank States - Temperature" <- w181
      }
      n183 = node-c288(w47) -> ()  [unwired: 1 out]
      n184 = xnode "Invoke Method"("FPGA VI Reference In"=w28) -> ()  [unwired: 1 in, 2 out]
      n185 = node-c288(w24) -> ()  [unwired: 1 out]
      n186 = node-c288(w45) -> ()  [unwired: 1 out]
      n187 = node-c288(w41) -> ()  [unwired: 1 out]
      n188 = node-c288(w49) -> ()  [unwired: 1 out]
      n189 = Merge Errors(w23, w22, w18, w19, w20) -> (w21:errorcluster)
    }
    frame #2 {
      # "Close"
      n190 = xnode "Close FPGA VI Reference"("FPGA VI Reference In"=w488, "error in"=w487) -> ("error out"=w486:errorcluster)
      n191 = call <vilib>:"Simple Error Handler.vi"("error in (no error)"=w486) -> ()  [unwired: 4 in, 5 out]
    }
  }
